vi "GUI.Config Test prueba con desplazador.vi"(11 "Path Config file":path) -> (3 "Path out":path)   [LabVIEW 2009]
uses:
  test.test de configuracion gui.ctl
  Test.ctl
  TEST.TEST CONFIG HW.ctl
  Rigol DP832/DP832_Control Channels.ctl
  TEST.TEST CONFIG TEST MATRIZ.ctl
  TEST.TEST CONFIG TEST.ctl
  TEST.TEST RESULT.ctl
  test_result fvasic.ctl
  TEST.TEST EXECUTION TEST.ctl
  TEST.TEST CONFIG VGA.ctl
  TEST.TEST TEST INFO.ctl
  TEST.TEST INFO PC.ctl
  machine estate configs.ctl
  Rigol DP832/DP832_Control Behavior.ctl
panel:
  out "FT_Handle":u32
  in  "Test":T1={"Config HW"={"VISA Rigol DP832"="Rigol_DP832", "Config Rigol DP832"=[{"Channel"=0, "V Limit"=5.5, "I Limit"=0.5, "V Out"=5.0}, {"Channel"=1, "V Limit"=5.5, "I Limit"=0.8, "V Out"=5.0}, {"Channel"=2, "V Limit"=5.5, "I Limit"=0.2, "V Out"=0.0}], "CTA Test#"="CTA013 A", "FT_Handle"=0, "Espera acceso FT"=10}, "Config Test"=[{"Vasic"=2.8, "Test Register?"=FALSE, "Test ADC?"=FALSE, "Test ADC"={"Repeats ADC"=100, "Max Desviation"=0.1}, "Limits ADC"={"Low"=[1.9, 1.3, 0.65, 0.0, 1.6, 1.4, 1.4, 0.9, 2.1, 0.85, 1.9], "High"=[2.1, 1.5, 0.85, 0.1, 1.4, 1.2, 1.2, 0.7, 1.9, 0.65, 1.7]}, "Test Max PN Min NP?"=FALSE, "Limits Max PN Min NP"={"Max P Upper"=1.888, "Min P Upper"=2.177000045776367, "Max N Upper"=0.818, "Min N Upper"=0.73, "Max P Lower"=1.475, "Min P Lower "=1.322, "Max N Lower"=1.321, "Min N Lower"=1.474}, "Test Rate Scan?"=FALSE, "Vin Rate Scan"=[], "Limits Rate Scan"={"High"=[0.15, 0.242, 0.331, 0.425, 0.512, 0.6, 0.688, 0.774, 0.847, 0.91], "Low"=[0.021, 0.11, 0.189, 0.27, 0.347, 0.421, 0.487, 0.551, 0.601, 0.635]}, "Test Rate Scan Adders?"=FALSE, "Vin Rate Adders"=[], "Test offset analog?"=FALSE, "Test offset digital?"=FALSE, "Lim Offset Analog"={"Max Analog"=0.05, "Min Analog"=-0.05}, "Lim offset Dig"={"Max Dig"=0.05}, "Limits Rate Scan adders"={"High"=[], "Low"=[]}}, {"Vasic"=2.8, "Test Register?"=FALSE, "Test ADC?"=FALSE, "Test ADC"={"Repeats ADC"=100, "Max Desviation"=0.1}, "Limits ADC"={"Low"=[1.9, 1.3, 0.65, 0.0, 1.6, 1.4, 1.4, 0.9, 2.1, 0.85, 1.9], "High"=[2.1, 1.5, 0.85, 0.1, 1.4, 1.2, 1.2, 0.7, 1.9, 0.65, 1.7]}, "Test Max PN Min NP?"=FALSE, "Limits Max PN Min NP"={"Max P Upper"=1.888, "Min P Upper"=2.177000045776367, "Max N Upper"=0.818, "Min N Upper"=0.73, "Max P Lower"=1.475, "Min P Lower "=1.322, "Max N Lower"=1.321, "Min N Lower"=1.474}, "Test Rate Scan?"=FALSE, "Vin Rate Scan"=[], "Limits Rate Scan"={"High"=[0.15, 0.242, 0.331, 0.425, 0.512, 0.6, 0.688, 0.774, 0.847, 0.91], "Low"=[0.021, 0.11, 0.189, 0.27, 0.347, 0.421, 0.487, 0.551, 0.601, 0.635]}, "Test Rate Scan Adders?"=FALSE, "Vin Rate Adders"=[], "Test offset analog?"=FALSE, "Test offset digital?"=FALSE, "Lim Offset Analog"={"Max Analog"=0.05, "Min Analog"=-0.05}, "Lim offset Dig"={"Max Dig"=0.05}, "Limits Rate Scan adders"={"High"=[], "Low"=[]}}, {"Vasic"=2.8, "Test Register?"=FALSE, "Test ADC?"=FALSE, "Test ADC"={"Repeats ADC"=100, "Max Desviation"=0.1}, "Limits ADC"={"Low"=[1.9, 1.3, 0.65, 0.0, 1.6, 1.4, 1.4, 0.9, 2.1, 0.85, 1.9], "High"=[2.1, 1.5, 0.85, 0.1, 1.4, 1.2, 1.2, 0.7, 1.9, 0.65, 1.7]}, "Test Max PN Min NP?"=FALSE, "Limits Max PN Min NP"={"Max P Upper"=1.888, "Min P Upper"=2.177000045776367, "Max N Upper"=0.818, "Min N Upper"=0.73, "Max P Lower"=1.475, "Min P Lower "=1.322, "Max N Lower"=1.321, "Min N Lower"=1.474}, "Test Rate Scan?"=FALSE, "Vin Rate Scan"=[], "Limits Rate Scan"={"High"=[0.15, 0.242, 0.331, 0.425, 0.512, 0.6, 0.688, 0.774, 0.847, 0.91], "Low"=[0.021, 0.11, 0.189, 0.27, 0.347, 0.421, 0.487, 0.551, 0.601, 0.635]}, "Test Rate Scan Adders?"=FALSE, "Vin Rate Adders"=[], "Test offset analog?"=FALSE, "Test offset digital?"=FALSE, "Lim Offset Analog"={"Max Analog"=0.05, "Min Analog"=-0.05}, "Lim offset Dig"={"Max Dig"=0.05}, "Limits Rate Scan adders"={"High"=[], "Low"=[]}}, {"Vasic"=2.8, "Test Register?"=FALSE, "Test ADC?"=FALSE, "Test ADC"={"Repeats ADC"=100, "Max Desviation"=0.1}, "Limits ADC"={"Low"=[1.9, 1.3, 0.65, 0.0, 1.6, 1.4, 1.4, 0.9, 2.1, 0.85, 1.9], "High"=[2.1, 1.5, 0.85, 0.1, 1.4, 1.2, 1.2, 0.7, 1.9, 0.65, 1.7]}, "Test Max PN Min NP?"=FALSE, "Limits Max PN Min NP"={"Max P Upper"=1.888, "Min P Upper"=2.177000045776367, "Max N Upper"=0.818, "Min N Upper"=0.73, "Max P Lower"=1.475, "Min P Lower "=1.322, "Max N Lower"=1.321, "Min N Lower"=1.474}, "Test Rate Scan?"=FALSE, "Vin Rate Scan"=[], "Limits Rate Scan"={"High"=[0.15, 0.242, 0.331, 0.425, 0.512, 0.6, 0.688, 0.774, 0.847, 0.91], "Low"=[0.021, 0.11, 0.189, 0.27, 0.347, 0.421, 0.487, 0.551, 0.601, 0.635]}, "Test Rate Scan Adders?"=FALSE, "Vin Rate Adders"=[], "Test offset analog?"=FALSE, "Test offset digital?"=FALSE, "Lim Offset Analog"={"Max Analog"=0.05, "Min Analog"=-0.05}, "Lim offset Dig"={"Max Dig"=0.05}, "Limits Rate Scan adders"={"High"=[], "Low"=[]}}], "Result"=[], "Execucion Test"={"Vasic Actual"=0}, "Config VGA"={"Theoretical Voltage"=[0.1, 0.2, 0.3, 0.4, 0.5, 0.6, 0.7, 0.8, 0.9, 1.0], "Real Voltage"=[0.10285, 0.20714, 0.29957, 0.40485, 0.49571, 0.60685, 0.69771, 0.80114, 0.89714, 0.99885], "Pulse Width"=57344, "Frecuency Pulse"=1000000.0, "VGA Gain"=[9, 16, 24, 34, 43, 52, 61, 72, 81, 93]}, "Test Info"={"Asic"="", "Operator"="", "Place"="", "Time start"=timestamp(0 s since 1904-01-01), "Time stop"=timestamp(0 s since 1904-01-01)}, "Info machine"={"SO"="", "SO Name"="", "SO Ver"="", "SO Build"="", "CPU"="", "APP"="", "APP YEAR"="", "APP ver"="", "APP User"="", "APP Serail"="", "MAC"=[], "PC NAME"=[], "PC IP"=[], "BIOS MANU"="", "BIOS NAME"="", "BIOS SERIAL"="", "BOARD MANU"="", "BOARD NAME"="", "BOARD SERIAL"="", "Driver Version"="", "Library Version"=""}} {"Config VGA"."Theoretical Voltage" format="%1.4f"; "Config VGA"."VGA Gain" format="%02x"; "Config VGA"."Frecuency Pulse" format="%0_2p"; "Config VGA"."Pulse Width" format="%04x"; "Config VGA"."Real Voltage" format="%1.5f"; "Config Test"."Limits Rate Scan adders"."Low" format="%1.3f"; "Config Test"."Limits Rate Scan adders"."High" format="%1.3f"; "Config Test"."Limits ADC"."High" format="%1.4f"; "Config Test"."Limits ADC"."Low" format="%1.3f"; "Config Test"."Lim offset Dig"."Max Dig" format="%.3g"; "Config Test"."Lim Offset Analog"."Min Analog" format="%.3g"; "Config Test"."Lim Offset Analog"."Max Analog" format="%.3g"; "Config Test"."Limits Rate Scan"."Low" format="%1.4f"; "Config Test"."Limits Rate Scan"."High" format="%1.3f"; "Config Test"."Limits Max PN Min NP"."Min P Upper" format="%.3g"; "Config Test"."Limits Max PN Min NP"."Min P Lower" format="%.3g"; "Config Test"."Limits Max PN Min NP"."Max N Lower" format="%.3g"; "Config Test"."Limits Max PN Min NP"."Max N Upper" format="%.3g"; "Config Test"."Limits Max PN Min NP"."Min N Lower" format="%.3g"; "Config Test"."Limits Max PN Min NP"."Min N Upper" format="%.3g"; "Config Test"."Limits Max PN Min NP"."Max P Upper" format="%.3g"; "Config Test"."Limits Max PN Min NP"."Max P Lower" format="%.3g"; "Config Test"."Vasic" min=2.8 max=3.8 step=0.01 format="%.2g"; "Config HW"."Config Rigol DP832"."Channel" items=["+30V Channel 1", "+30V Channel 2", "+5V Channel 3"]; "Config HW"."Config Rigol DP832"."V Limit" format="%.1g"; "Config HW"."Config Rigol DP832"."I Limit" format="%.1g"; "Config HW"."Config Rigol DP832"."V Out" format="%.1g"; "Result"."Test Registros"."Read W/R" format="%04x"; "Result"."Test Registros"."Pattern W/R" format="%04x"; "Result"."Test Registros"."Read Default" format="%04x"; "Result"."Test Registros"."Pattern Default" format="%04x"}
  in  "visualize":enum32{"Page 1", "Page 2"}(tab)
  in  "Elemensts":i32(listbox)
  in  "vga test":T12={"FRECUENCY PULSE"=-0.05, "PULSE WIDTH"=0, "CODE GAIN TEST"=0} {"CODE GAIN TEST" max=127 step=1; "PULSE WIDTH" format="%04x"; "FRECUENCY PULSE" format="%.3p"}
  in  "CTA Board":string(combo)
  in  "CHECK vga":bool
  in  "CHECK cta":bool
  in  "CHECK POWER":bool
  in  "Config Rigol DP832":T13(array[cluster])=[{"Channel"=0, "V Limit"=5.5, "I Limit"=0.5, "V Out"=5.0}, {"Channel"=1, "V Limit"=5.5, "I Limit"=0.8, "V Out"=5.0}, {"Channel"=2, "V Limit"=5.5, "I Limit"=0.2, "V Out"=0.0}] {"Channel" items=["+30V Channel 1", "+30V Channel 2", "+5V Channel 3"]; "V Limit" min=0.0 max=6.0 step=0.1 format="%.1g"; "I Limit" min=0.0 max=1.0 step=0.1 format="%.1g"; "V Out" min=0.0 max=6.0 step=0.1 format="%.1g"}
  in  "copy to new":bool
  in  "new":bool
  in  "delete":bool
  in  "TEST#":i32
  in  "VGA":T14={"VALUES VGA"=[], "TIME VGA"={"PULSE WIDTH"=0, "FRECUENCY PULSE"=-0.05}} {"TIME VGA"."FRECUENCY PULSE" format="%.3p"; "TIME VGA"."PULSE WIDTH" format="%04x"}
  in  "Valores":T15[](array[typedef])=[{"VOLTAGE SUPPLY ASIC"=2.5, "TEST ADC"=FALSE, "SETUP ADC 2"={"NUMBER OF REPETITIONS"=0, "MAX DESVIATION ADC"=-0.05}, "LIMITS MEASUREMENT ADC"=[], "TEST MAX MIN P/N"=FALSE, "LIMITS MAX PN MIN NP"=[], "TEST RATE SCAN"=FALSE, "VIN ASIC"=[], "LIMITS RATE SCAN"=[], "TEST RATE SCAN ADDERS"=FALSE, "VIN ASIC ADD"=[], "LIMITS RATE SCAN ADDERS"=[], "TEST OFFSET ANALOG"=FALSE, "LIMITS OFFSET ANALOG"={"MAXIMUM"=0.05, "MINIMUM"=-0.05}, "TEST OFFSET DIGITAL"=FALSE, "LIMITS OFFSET DIGITAL"={"MAXIMUM"=0.05}, "TEST REGISTER"=FALSE}] {"VOLTAGE SUPPLY ASIC" min=2.5 max=3.5 step=0.1 format="%.2g"; "LIMITS OFFSET DIGITAL"."MAXIMUM" format="%.3g"; "LIMITS OFFSET ANALOG"."MINIMUM" format="%.3g"; "LIMITS OFFSET ANALOG"."MAXIMUM" format="%.3g"; "SETUP ADC 2"."MAX DESVIATION ADC" format="%.3g"}
  in  "default":bool
  in  "Load config":bool
  in  "save config":bool
  in  "QUIT":bool
  in  "VISA Rigol DP832":refnum<visa-resource-name>="Rigol_DP832"
  # "Modo 2\nModo 3\nModo 4\nModo 2\nModo 3\nModo 4"
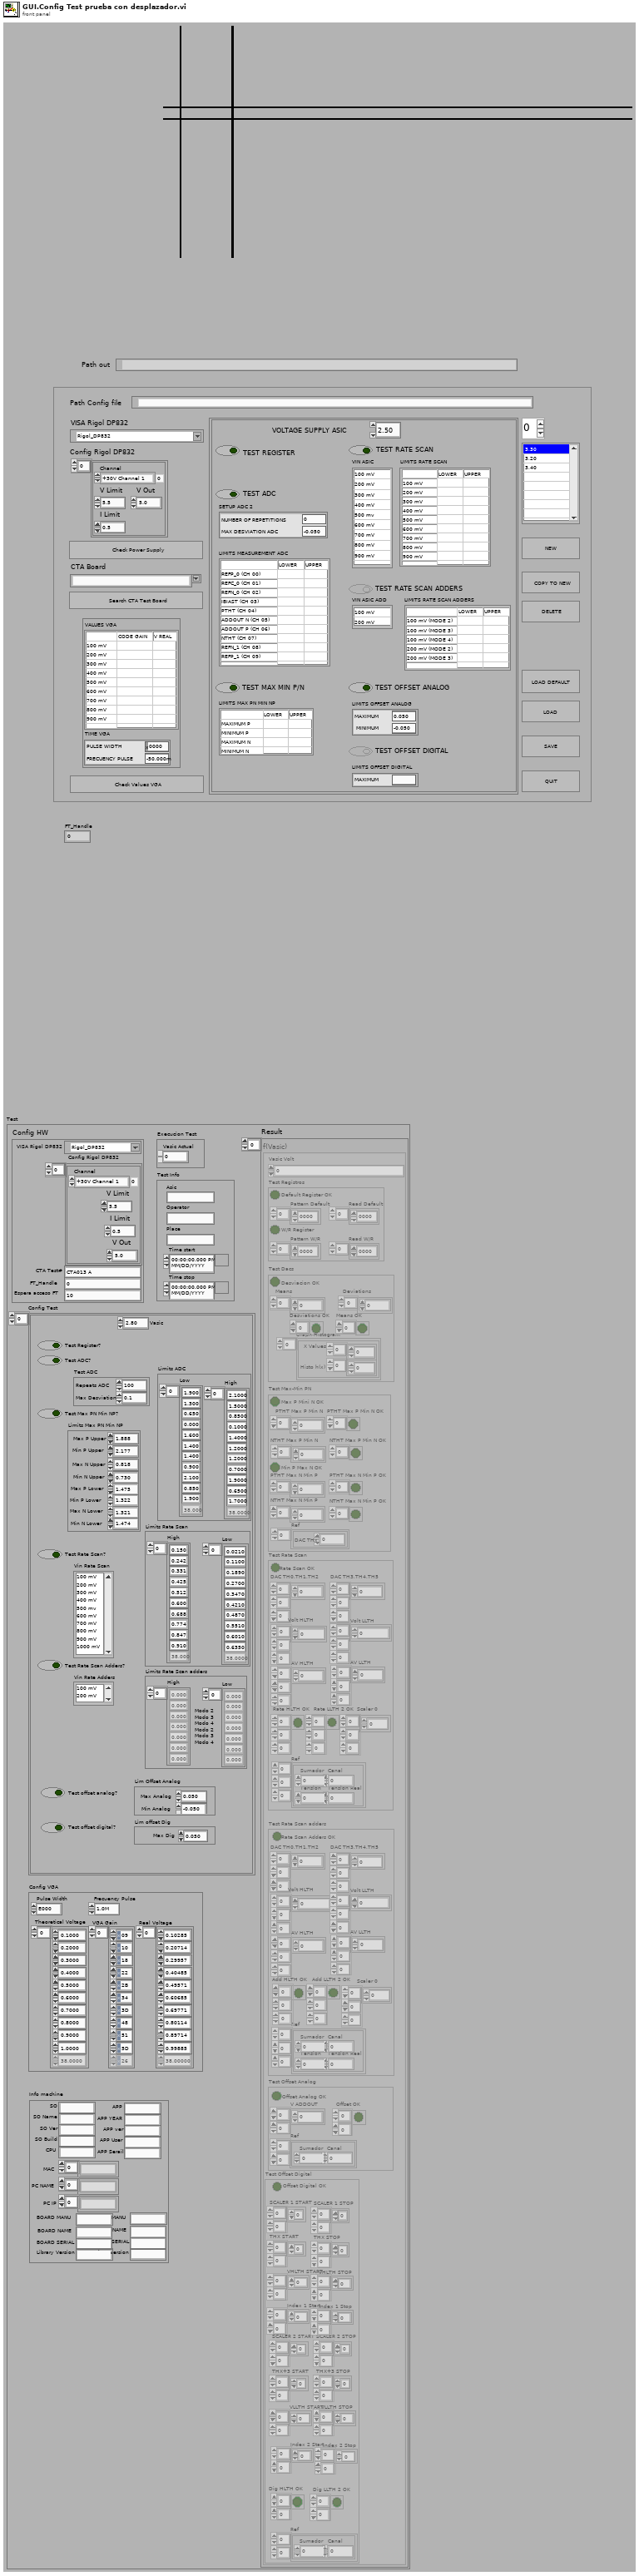
[diagram p1: front panel]
types:
  T1 = typedef "Test.ctl" = cluster{"Config HW":T2, "Config Test":T4, "Result":T6, "Execucion Test":T8, "Config VGA":T9, "Test Info":T10, "Info machine":T11}
  T2 = typedef "TEST.TEST CONFIG HW.ctl" = cluster{"VISA Rigol DP832":refnum<visa-resource-name>, "Config Rigol DP832":cluster{"Channel":T3, "V Limit":dbl, "I Limit":dbl, "V Out":dbl}[], "CTA Test#":string, "FT_Handle":u32, "Espera acceso FT":u32}
  T3 = typedef "DP832_Control Channels.ctl" = i32
  T4 = typedef "TEST.TEST CONFIG TEST MATRIZ.ctl" = T5[]
  T5 = typedef "TEST.TEST CONFIG TEST.ctl" = cluster{"Vasic":dbl, "Test Register?":bool, "Test ADC?":bool, "Test ADC":cluster{"Repeats ADC":i32, "Max Desviation":dbl}, "Limits ADC":cluster{"Low":dbl[], "High":dbl[]}, "Test Max PN Min NP?":bool, "Limits Max PN Min NP":cluster{"Max P Upper":dbl, "Min P Upper":dbl, "Max N Upper":dbl, "Min N Upper":dbl, "Max P Lower":dbl, "Min P Lower ":dbl, "Max N Lower":dbl, "Min N Lower":dbl}, "Test Rate Scan?":bool, "Vin Rate Scan":i32[], "Limits Rate Scan":cluster{"High":dbl[], "Low":dbl[]}, "Test Rate Scan Adders?":bool, "Vin Rate Adders":i32[], "Test offset analog?":bool, "Test offset digital?":bool, "Lim Offset Analog":cluster{"Max Analog":dbl, "Min Analog":dbl}, "Lim offset Dig":cluster{"Max Dig":dbl}, "Limits Rate Scan adders":cluster{"High":dbl[], "Low":dbl[]}}
  T6 = typedef "TEST.TEST RESULT.ctl" = T7[]
  T7 = typedef "test_result fvasic.ctl" = cluster{"Vasic Volt":i32, "Test Registros":cluster{"Default Register OK":bool, "Pattern Default":u16[], "Read Default":u16[], "W/R Register":bool, "Pattern W/R":u16[], "Read W/R":u16[]}, "Test Dacs":cluster{"Desviacion OK":bool, "Means":dbl[], "Deviations":dbl[], "Desviations OK":bool[], "Means OK":bool[], "Graph Histogram":cluster{"X Values":dbl[], "Histo h(x)":i32[]}[]}, "Test Max-Min PN":cluster{"Max P Mini N OK":bool, "PTHT Max P Min N":dbl[], "PTHT Max P Min N OK":bool[], "NTHT Max P Min N":dbl[], "NTHT Max P Min N OK":bool[], "Min P Max N OK":bool, "PTHT Max N Min P":dbl[], "PTHT Max N Min P OK":bool[], "NTHT Max N Min P":dbl[], "NTHT Max N Min P OK":bool[], "Ref":cluster{"DAC THx":u8}[]}, "Test Rate Scan":cluster{"Rate Scan OK":bool, "DAC TH0,TH1,TH2":u16[][][], "Volt HLTH":dbl[][][], "AV HLTH":dbl[][][], "Rate HLTH OK":bool[][][], "DAC TH3,TH4,TH5":u16[][][], "Volt LLTH":dbl[][][], "AV LLTH":dbl[][][], "Rate LLTH 2 OK":bool[][][], "Scaler 0":u16[][][], "Ref":cluster{"Sumador":u8, "Canal":u8, "Tension":u8, "Tension Real":dbl}[][][]}, "Test Rate Scan adders":cluster{"Rate Scan Adders OK":bool, "DAC TH0,TH1,TH2":u16[][][], "Volt HLTH":dbl[][][], "AV HLTH":dbl[][][], "Add HLTH OK":bool[][][], "DAC TH3,TH4,TH5":u16[][][], "Volt LLTH":dbl[][][], "AV LLTH":dbl[][][], "Add LLTH 2 OK":bool[][][], "Scaler 0":u16[][][], "Ref":cluster{"Sumador":u8, "Canal":u8, "Tension":u8, "Tension Real":dbl}[][][]}, "Test Offset Analog":cluster{"Offset Analog OK":bool, "V ADDOUT":dbl[][], "Offset OK":bool[][], "Ref":cluster{"Sumador":u8, "Canal":u8}[][]}, "Test Offset Digital":cluster{"Offset Digital OK":bool, "SCALER 1 START":u16[][], "SCALER 1 STOP":u16[][], "THX START":u16[][], "THX STOP":u16[][], "VHLTH START":dbl[][], "VHLTH STOP":dbl[][], "Index 1 Start":i32[][], "index 1 Stop":i32[][], "SCALER 2 START":u16[][], "SCALER 2 STOP":u16[][], "THX+3 START":u16[][], "THX+3 STOP":u16[][], "VLLTH START":dbl[][], "VLLTH STOP":dbl[][], "Index 2 Start":i32[][], "index 2 Stop":i32[][], "Dig HLTH OK":bool[][], "Dig LLTH 2 OK":bool[][], "Ref":cluster{"Sumador":u8, "Canal":u8}[][]}}
  T8 = typedef "TEST.TEST EXECUTION TEST.ctl" = cluster{"Vasic Actual":i32}
  T9 = typedef "TEST.TEST CONFIG VGA.ctl" = cluster{"Theoretical Voltage":dbl[], "Real Voltage":dbl[], "Pulse Width":u16, "Frecuency Pulse":dbl, "VGA Gain":u8[]}
  T10 = typedef "TEST.TEST TEST INFO.ctl" = cluster{"Asic":string, "Operator":string, "Place":string, "Time start":timestamp, "Time stop":timestamp}
  T11 = typedef "TEST.TEST INFO PC.ctl" = cluster{"SO":string, "SO Name":string, "SO Ver":string, "SO Build":string, "CPU":string, "APP":string, "APP YEAR":string, "APP ver":string, "APP User":string, "APP Serail":string, "MAC":string[], "PC NAME":string[], "PC IP":string[], "BIOS MANU":string, "BIOS NAME":string, "BIOS SERIAL":string, "BOARD MANU":string, "BOARD NAME":string, "BOARD SERIAL":string, "Driver Version":string, "Library Version":string}
  T12 = cluster{"FRECUENCY PULSE":dbl, "PULSE WIDTH":u16, "CODE GAIN TEST":u8}
  T13 = cluster{"Channel":T3, "V Limit":dbl, "I Limit":dbl, "V Out":dbl}[]
  T14 = cluster{"VALUES VGA":string[][], "TIME VGA":cluster{"PULSE WIDTH":u16, "FRECUENCY PULSE":dbl}}
  T15 = typedef "test.test de configuracion gui.ctl" = cluster{"VOLTAGE SUPPLY ASIC":dbl, "TEST ADC":bool, "SETUP ADC 2":cluster{"NUMBER OF REPETITIONS":i32, "MAX DESVIATION ADC":dbl}, "LIMITS MEASUREMENT ADC":string[][], "TEST MAX MIN P/N":bool, "LIMITS MAX PN MIN NP":string[][], "TEST RATE SCAN":bool, "VIN ASIC":i32[], "LIMITS RATE SCAN":string[][], "TEST RATE SCAN ADDERS":bool, "VIN ASIC ADD":i32[], "LIMITS RATE SCAN ADDERS":string[][], "TEST OFFSET ANALOG":bool, "LIMITS OFFSET ANALOG":cluster{"MAXIMUM":dbl, "MINIMUM":dbl}, "TEST OFFSET DIGITAL":bool, "LIMITS OFFSET DIGITAL":cluster{"MAXIMUM":dbl}, "TEST REGISTER":bool}
  T16 = typedef "machine estate configs.ctl" = enum16{"Init", "load init file", "wait", "Load File", "Refresh", "quit", "Save File", "Valores>Test", "Test>View", "quit save"}
  T17 = enum8{"Enabled", "Disabled", "Disabled and Grayed Out"}
  T18 = cluster{"VOLTAGE SUPPLY ASIC":dbl, "TEST ADC":bool, "SETUP ADC 2":cluster{"NUMBER OF REPETITIONS":i32, "MAX DESVIATION ADC":dbl}, "LIMITS MEASUREMENT ADC":string[][], "TEST MAX MIN P/N":bool, "LIMITS MAX PN MIN NP":string[][], "TEST RATE SCAN":bool, "VIN ASIC":i32[], "LIMITS RATE SCAN":string[][], "TEST RATE SCAN ADDERS":bool, "VIN ASIC ADD":i32[], "LIMITS RATE SCAN ADDERS":string[][], "TEST OFFSET ANALOG":bool, "LIMITS OFFSET ANALOG":cluster{"MAXIMUM":dbl, "MINIMUM":dbl}, "TEST OFFSET DIGITAL":bool, "LIMITS OFFSET DIGITAL":cluster{"MAXIMUM":dbl}, "TEST REGISTER":bool}[]
  T19 = cluster{"CTA Test#":string, "CTA Test#":string}[]
  T20 = cluster{"VISA Rigol DP832":refnum<visa-resource-name>, "CTA Test#":string}
  T21 = cluster{"Vsupply asic":dbl, "Test Register??":bool, "Test ADC??":bool, "Test ADC set":cluster{"Repeats ADC":i32, "Max Desviation":dbl}, "High ADC means":dbl[], "Low ADC means":dbl[], "Test MAX/MIN??":bool, "Limits Max PN Min NP":cluster{"Max P Lower":dbl, "Min P Lower ":dbl, "Max N Lower":dbl, "Min N Lower":dbl, "Max P Upper":dbl, "Min P Upper":dbl, "Min N Upper":dbl, "Max N Upper":dbl}, "Test rate scan":bool, "Vin Rate Scan":i32[], "High rate scan":dbl[], "Low rate scan":dbl[], "Test rate scan adders??":bool, "Vin Rate Adders":i32[], "High rate scan add":dbl[], "Low rate scan add":dbl[], "Test offset analog??":bool, "Lim Offset Analog":cluster{"Max Analog":dbl, "Min Analog":dbl}, "Test offset digital??":bool, "Lim offset Dig":cluster{"Max Dig":dbl}}[]
  T22 = typedef "DP832_Control Behavior.ctl" = u16
  T23 = cluster{"Device Index":u32, "FT_FLAGS_OPENED":bool, "FT_FLAGS_HISPEED":bool, "Type":u32, "VID":u32, "PID":u32, "LocID":i32, "Serial Number":string, "Description":string, "FT_Handle":u32}[]
  T24 = cluster{"Device Index":u32, "FT_FLAGS_OPENED":bool, "FT_FLAGS_HISPEED":bool, "Type":u32, "VID":u32, "PID":u32, "LocID":i32, "Serial Number":string, "Description":string, "FT_Handle":u32}
  T25 = cluster{"Serial Number":string, "Serial Number":string}
  T26 = cluster{"Vsupply asic":dbl, "Test Register??":bool, "Test ADC??":bool, "Test ADC set":cluster{"Repeats ADC":i32, "Max Desviation":dbl}, "High ADC means":dbl[], "Low ADC means":dbl[], "Test MAX/MIN??":bool, "Limits Max PN Min NP":cluster{"Max P Lower":dbl, "Min P Lower ":dbl, "Max N Lower":dbl, "Min N Lower":dbl, "Max P Upper":dbl, "Min P Upper":dbl, "Min N Upper":dbl, "Max N Upper":dbl}, "Test rate scan":bool, "Vin Rate Scan":i32[], "High rate scan":dbl[], "Low rate scan":dbl[], "Test rate scan adders??":bool, "Vin Rate Adders":i32[], "High rate scan add":dbl[], "Low rate scan add":dbl[], "Test offset analog??":bool, "Lim Offset Analog":cluster{"Max Analog":dbl, "Min Analog":dbl}, "Test offset digital??":bool, "Lim offset Dig":cluster{"Max Dig":dbl}}
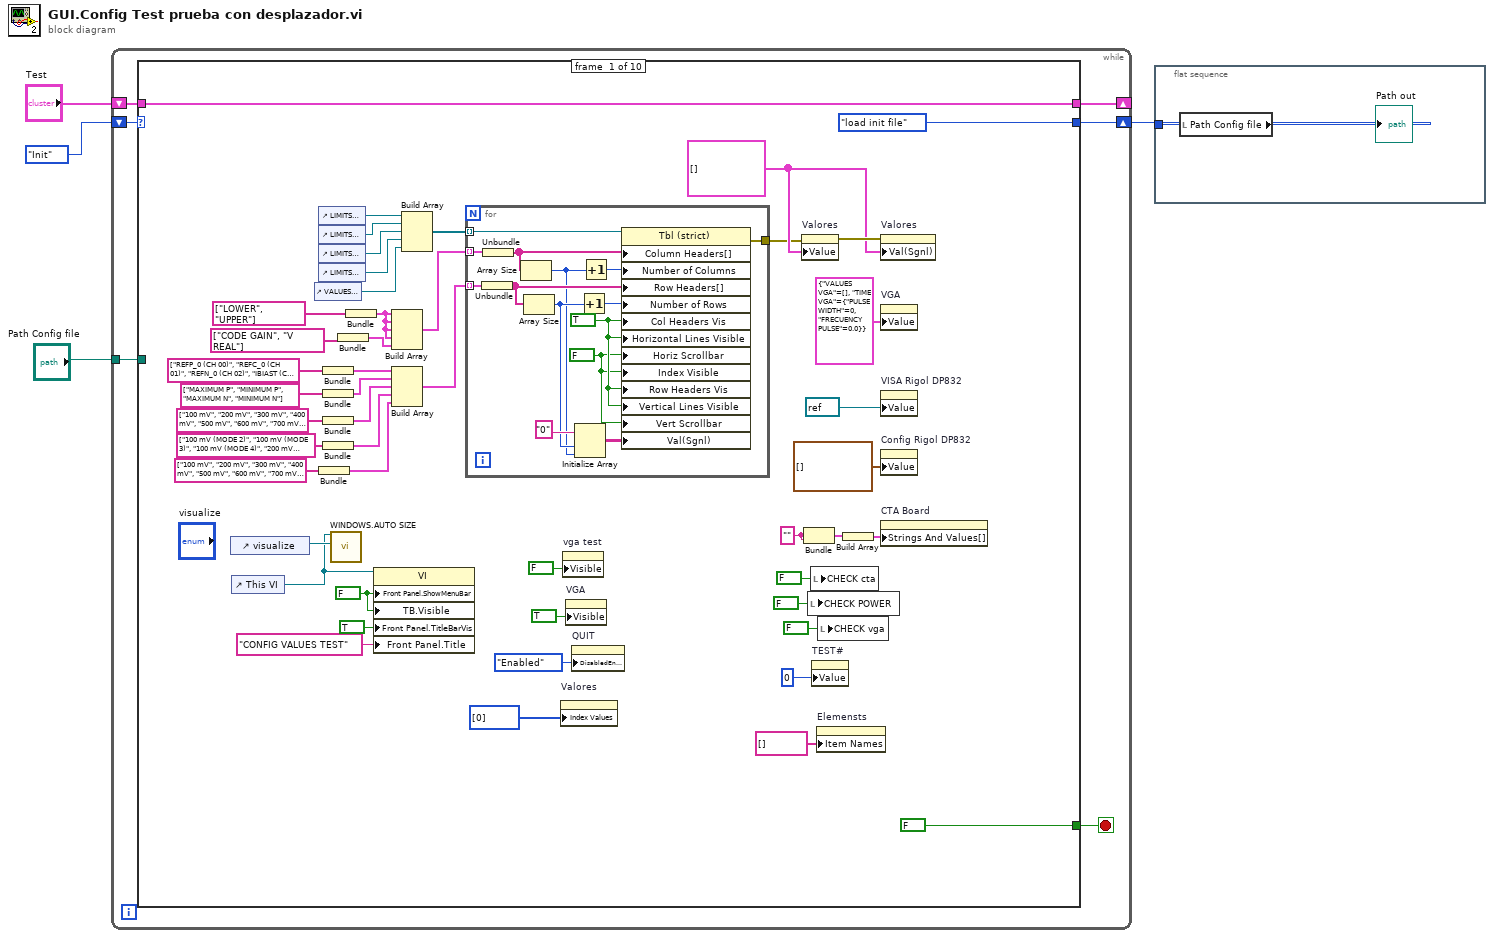
[diagram p0: block diagram]
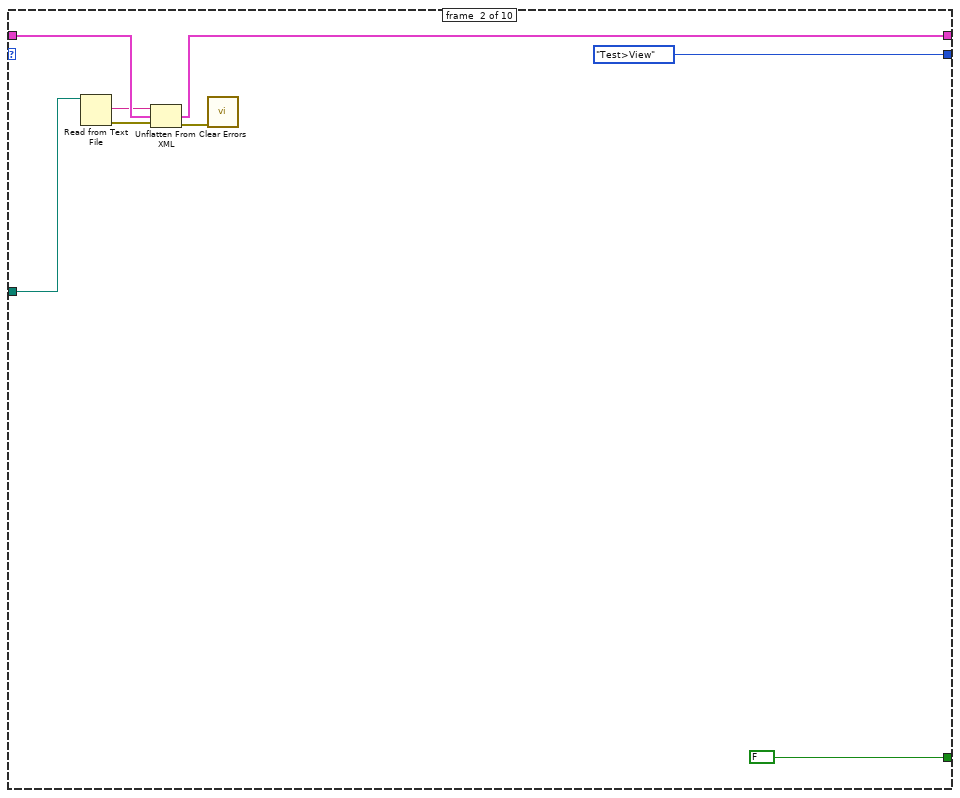
[diagram p2: hidden frame]
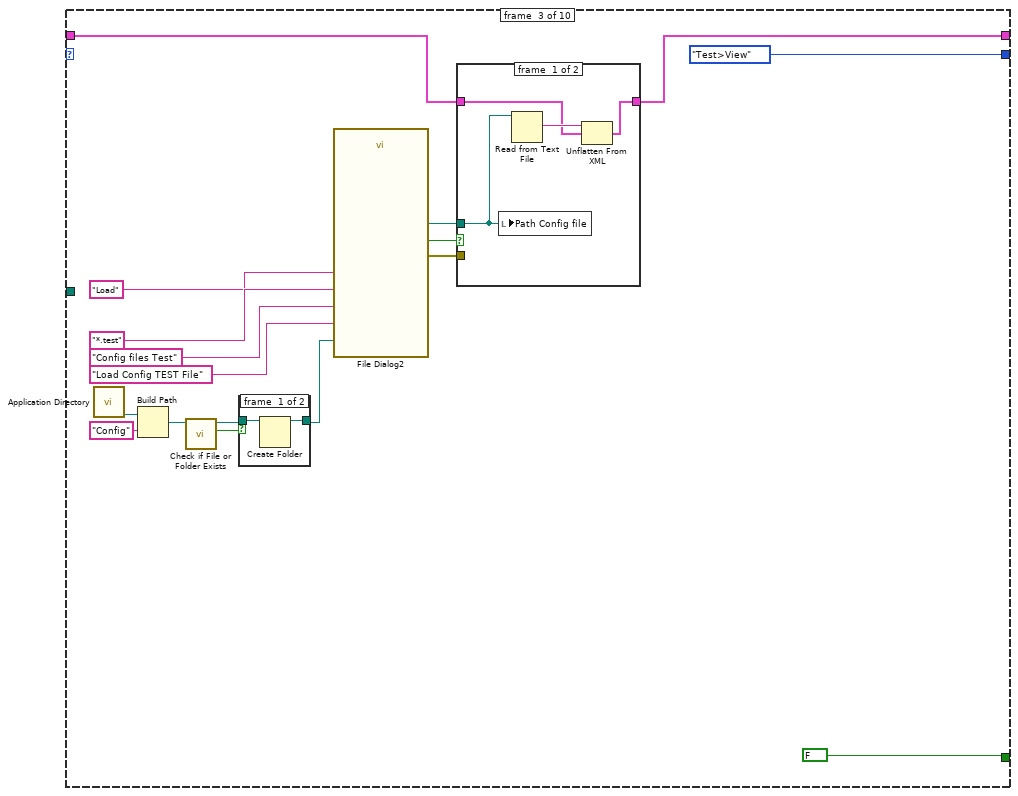
[diagram p3: hidden frame]
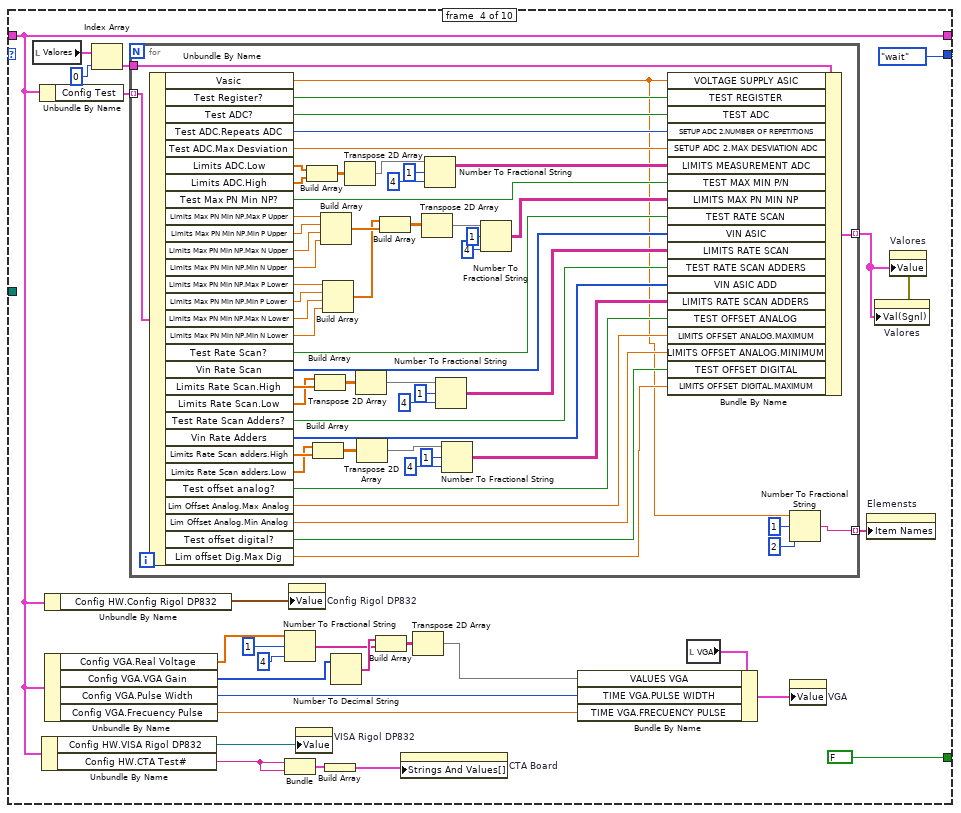
[diagram p6: hidden frame]
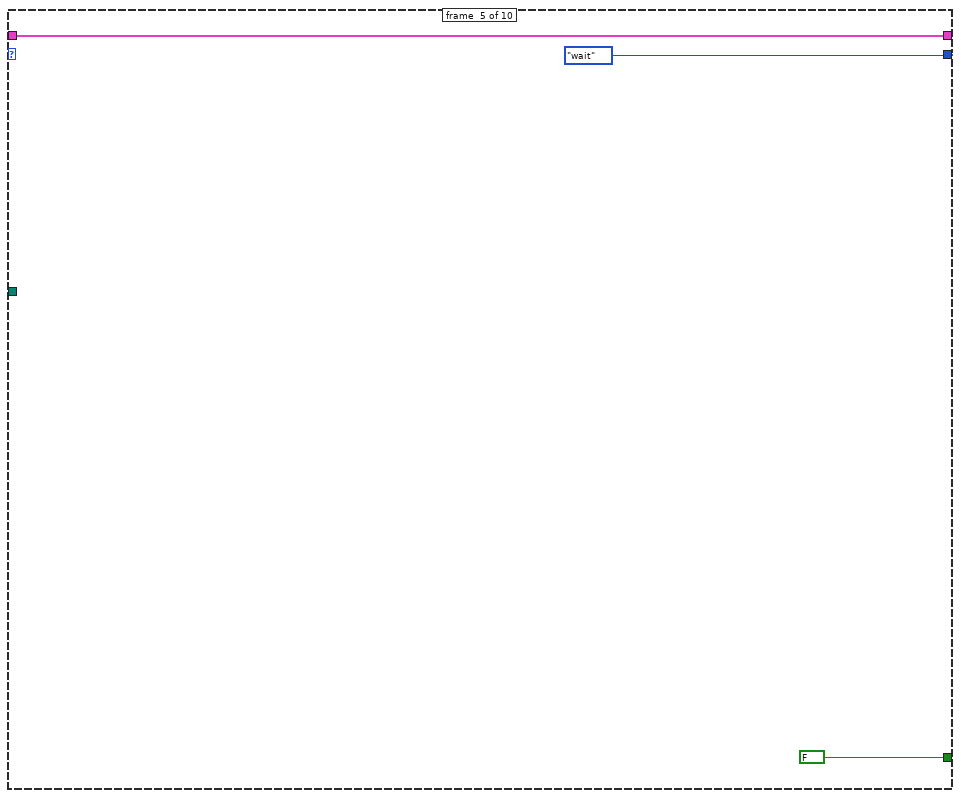
[diagram p7: hidden frame]
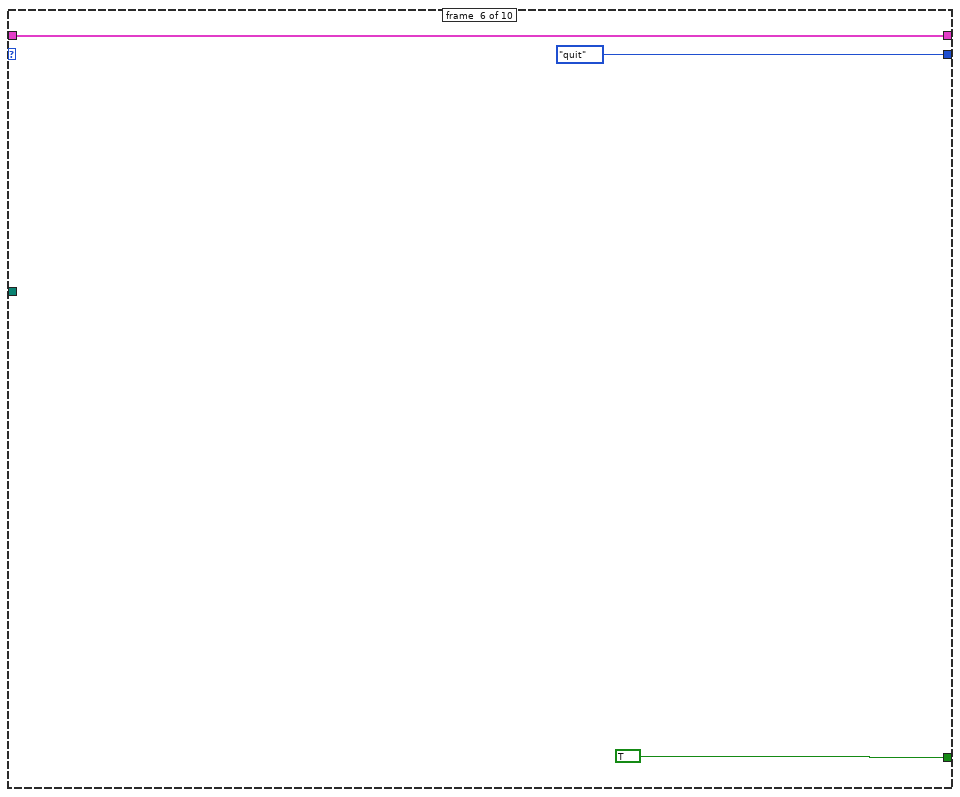
[diagram p8: hidden frame]
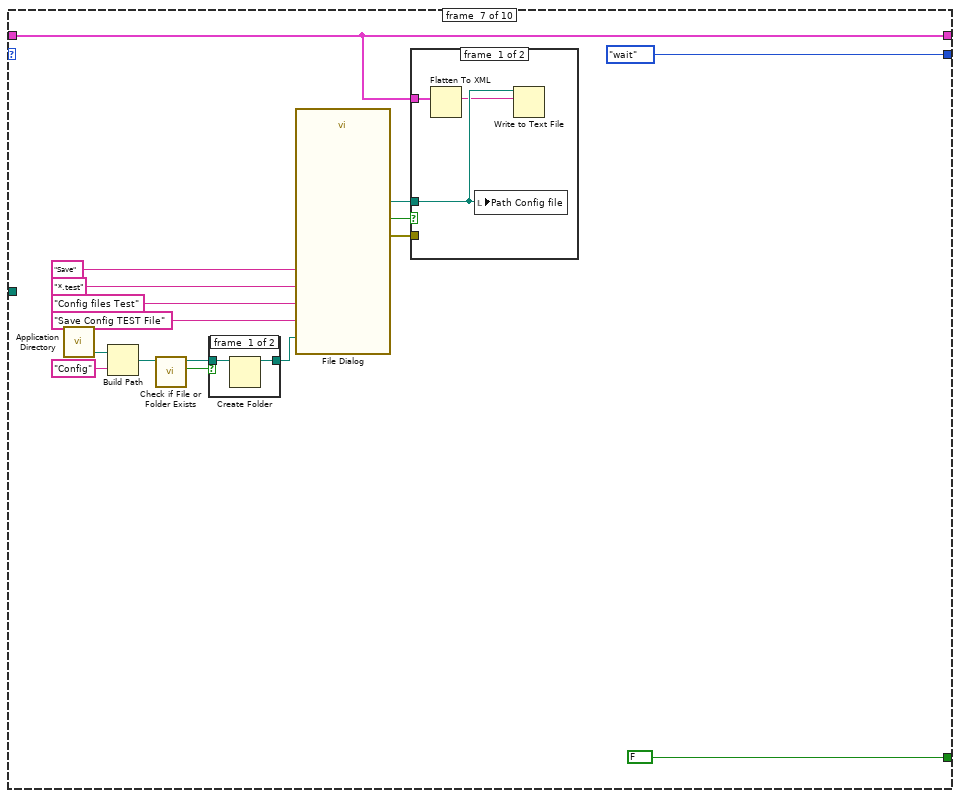
[diagram p9: hidden frame]
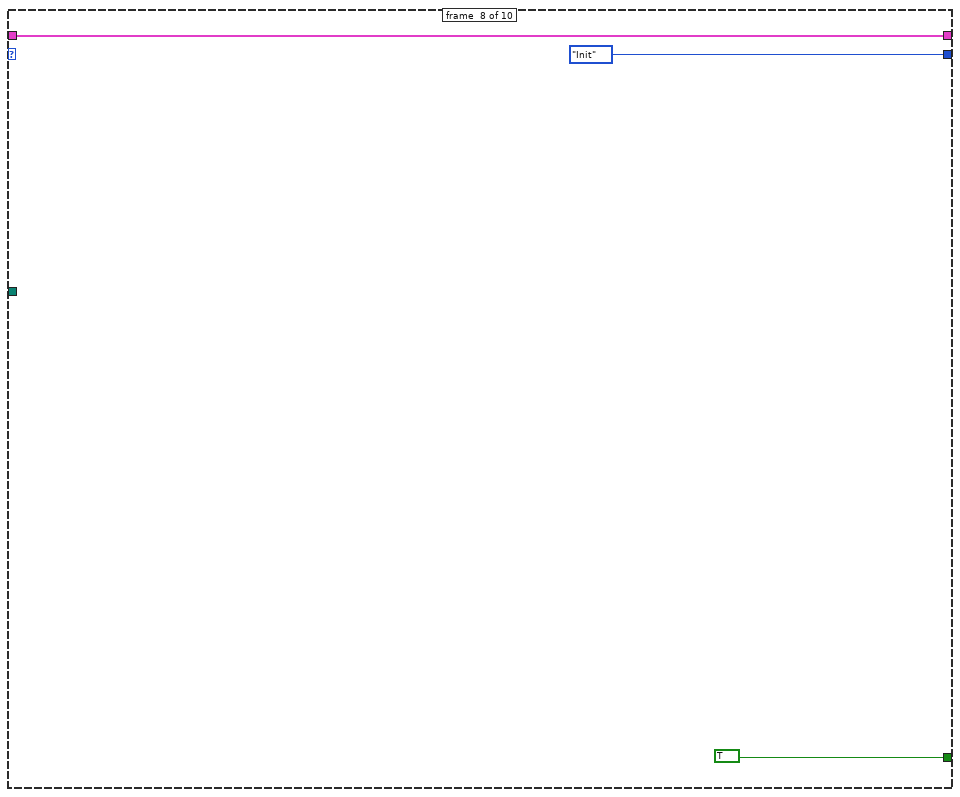
[diagram p12: hidden frame]
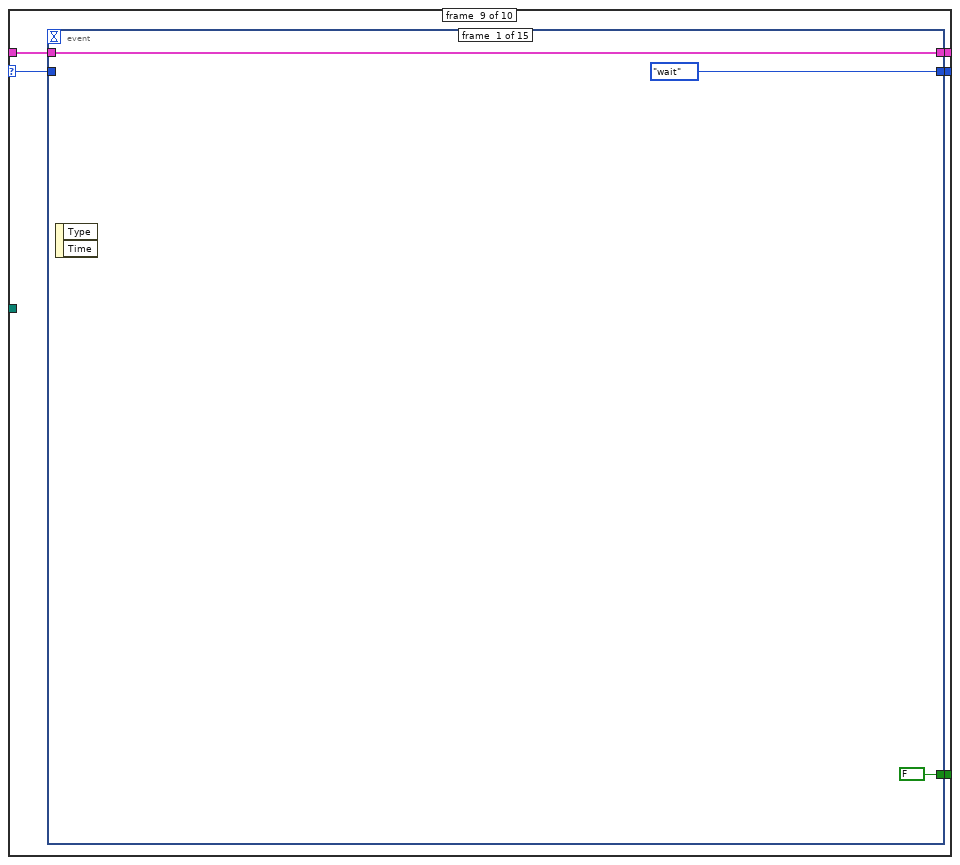
[diagram p13: hidden frame]
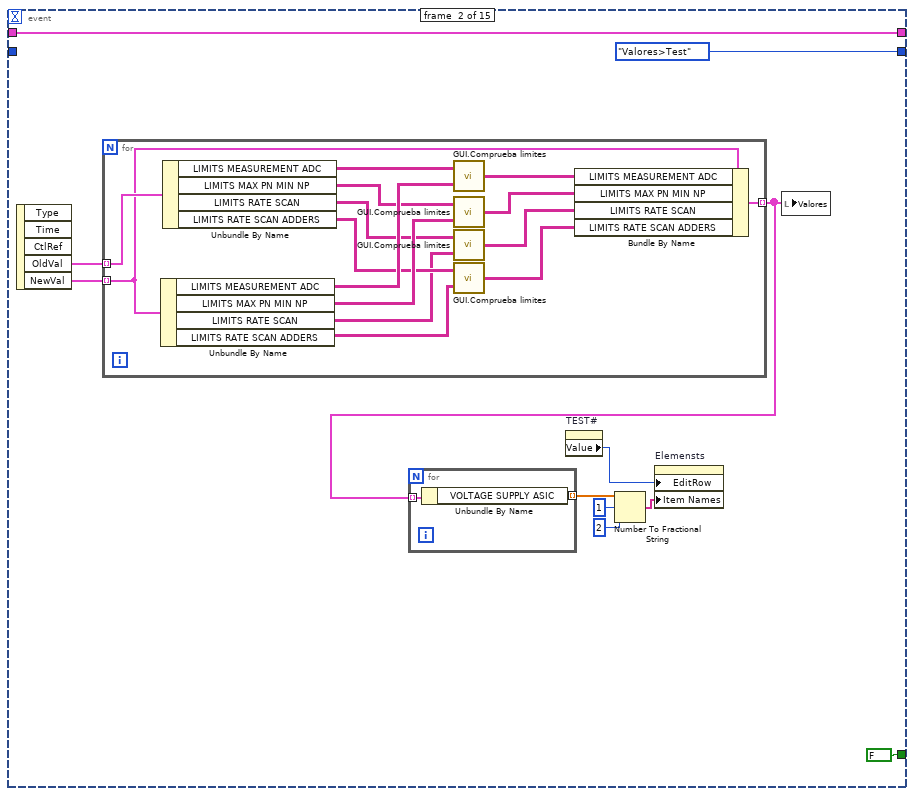
[diagram p14: hidden frame]
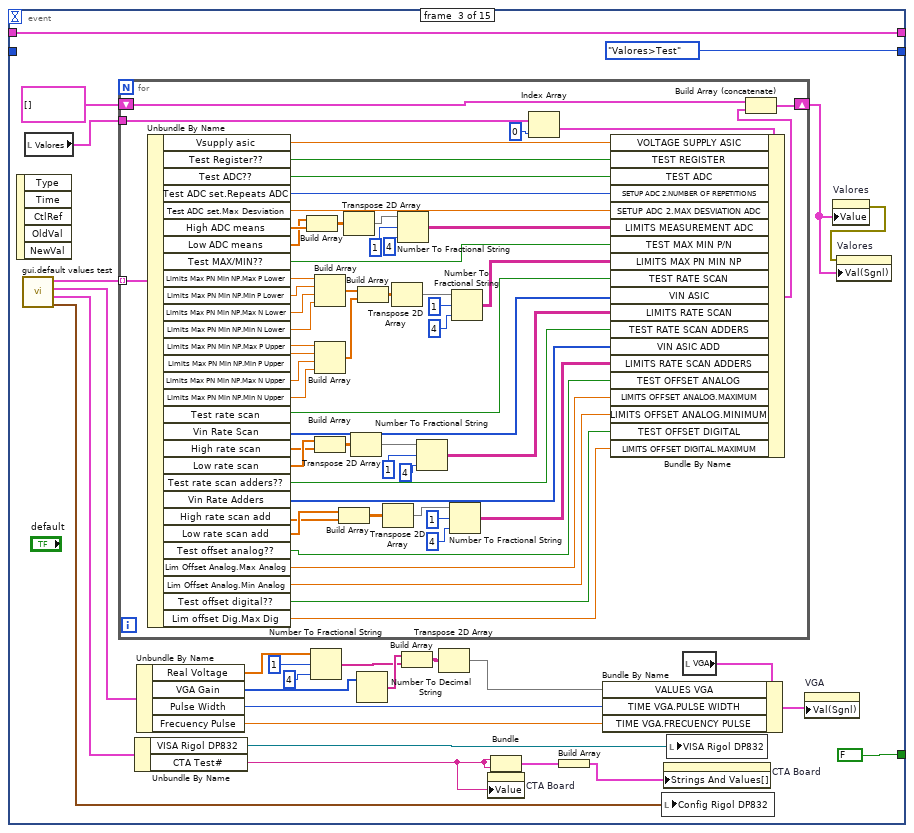
[diagram p15: hidden frame]
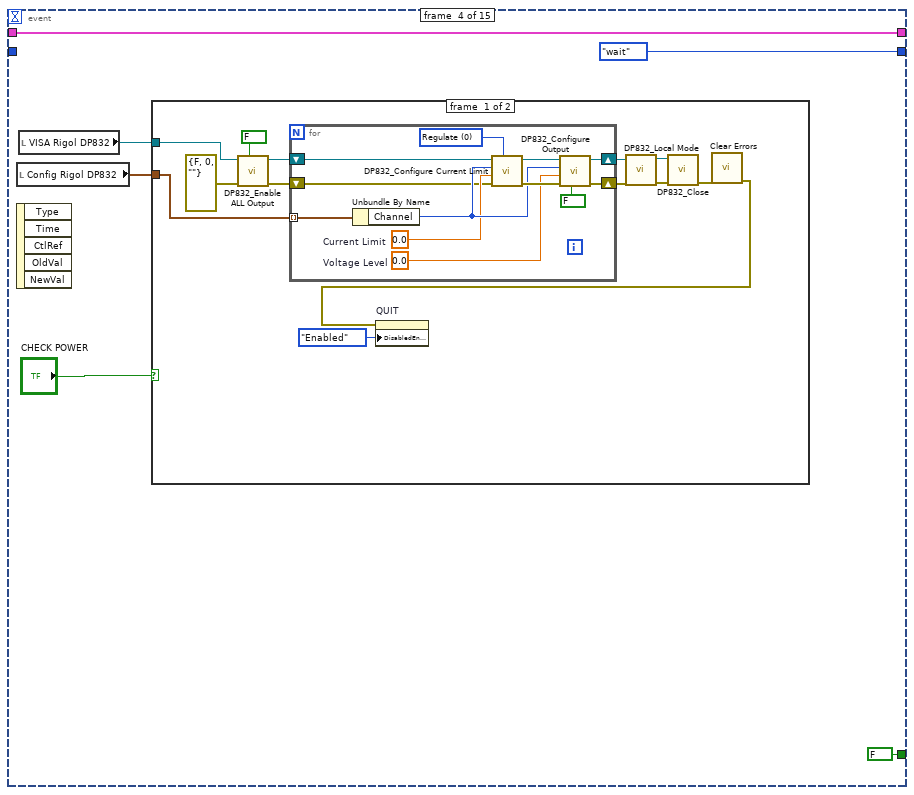
[diagram p16: hidden frame]
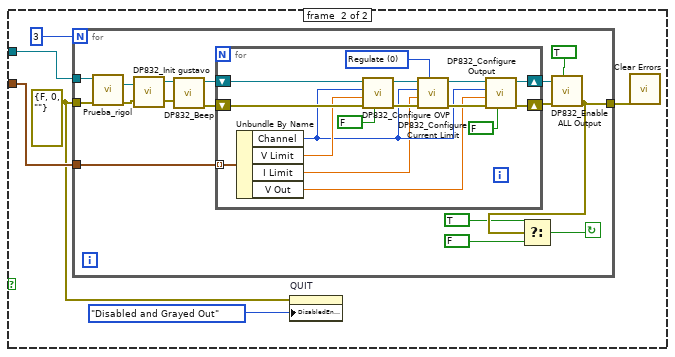
[diagram p17: hidden frame]
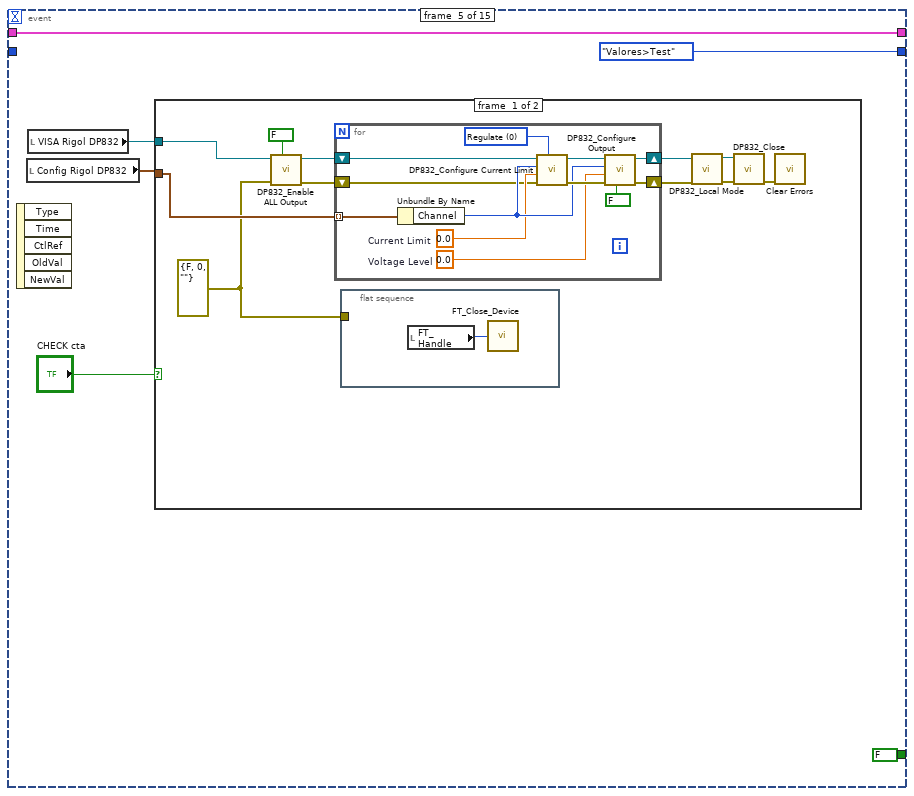
[diagram p18: hidden frame]
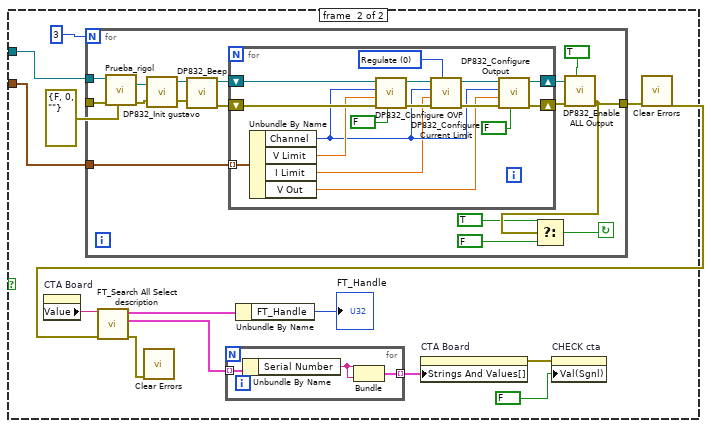
[diagram p19: hidden frame]
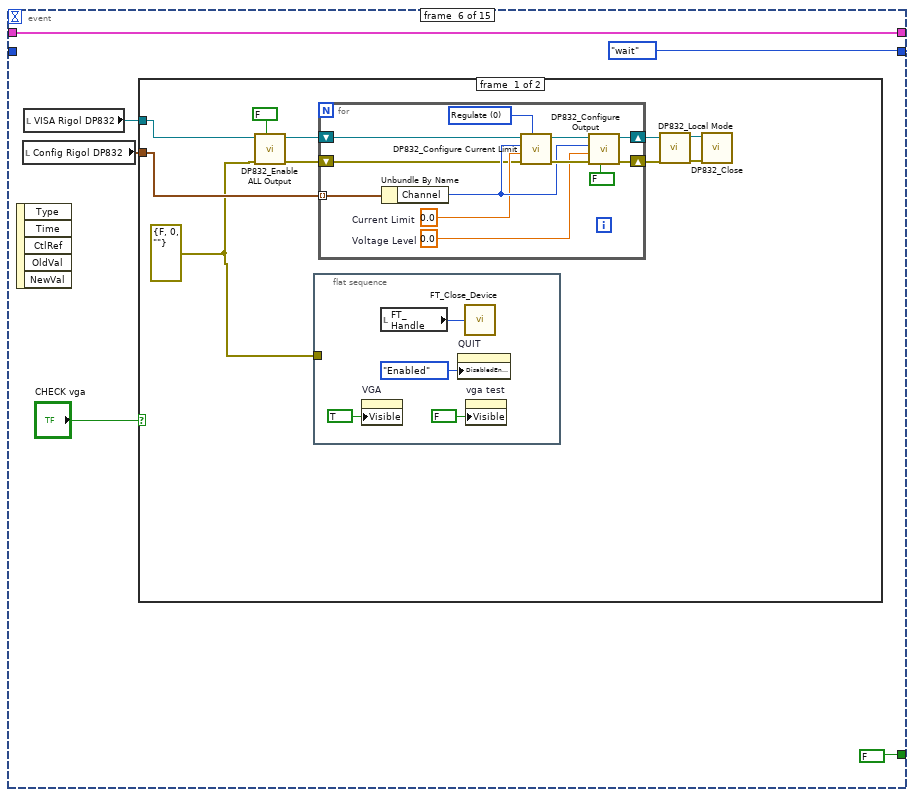
[diagram p20: hidden frame]
diagram:
  n1 = while {
    shift-right: [w8] -> w1
    shift-left: machine_estate_configs."Init" ("MACHINE") -> [w9]
    shift-right: [w6] -> _
    shift-left: "Test" -> [w7]
    tunnel: "Path Config file" -> [w5]
    stop <- w10 stop-if-true
    n2 = case shown="\"wait\"" w9 {
      selector: w9 -> [_ _ _ _ _ _ _ _ w224 _]
      tunnel: [FALSE FALSE FALSE FALSE FALSE TRUE FALSE TRUE w225 FALSE] -> w10
      tunnel: [machine_estate_configs."load init file" ("MACHINE") machine_estate_configs."Test>View" ("MACHINE") machine_estate_configs."Test>View" ("MACHINE") machine_estate_configs."wait" ("MACHINE") machine_estate_configs."wait" ("MACHINE") machine_estate_configs."quit" ("MACHINE") machine_estate_configs."wait" ("MACHINE") machine_estate_configs."Init" ("MACHINE") w223 machine_estate_configs."wait" ("MACHINE")] -> w8
      tunnel: [w29 w79 w82 w111 w190 w193 w196 w218 w221 w821] -> w6
      tunnel: w7 -> [w29 w80 w83 w111 w190 w193 w196 w218 w222 w822]
      tunnel: w5 -> [_ w75 _ _ _ _ _ _ _ _]
      frame #0 {
        w25 = T15[] [] ("Valores")
        w19 = "" ("CTA Test#")
        w41 = FALSE ("Front Panel Window:Show Menu Bar")
        n3 = control-ref of="visualize"() -> (w56:refnum<vi>)
        n4 = control-ref of="This VI"() -> (w38:refnum<vi>)
        n5 = control-ref of="VALUES VGA"() -> (w37:refnum<vi>)
        n6 = control-ref of="LIMITS MEASUREMENT ADC"() -> (w55:refnum<vi>)
        n7 = control-ref of="LIMITS MAX PN MIN NP"() -> (w54:refnum<vi>)
        n8 = control-ref of="LIMITS RATE SCAN"() -> (w53:refnum<vi>)
        n9 = control-ref of="LIMITS RATE SCAN ADDERS"() -> (w52:refnum<vi>)
        n10 = Bundle("Column Headers"=string[] ["100 mV", "200 mV", "300 mV", "400 mV", "500 mV", "600 mV", "700 mV", "800 mV", "900 mV", "1000 mV"]) -> (w32:cluster{"Column Headers":string[]})  [unwired: 1 in]
        n11 = Bundle("Column Headers"=string[] ["REFP_0 (CH 00)", "REFC_0 (CH 01)", "REFN_0 (CH 02)", "IBIAST (CH 03)", "PTHT (CH 04)", "ADDOUT N (CH 05)", "ADDOUT P (CH 06)", "NTHT (CH 07)", "REFN_1 (CH 08)", "REFP_1 (CH 09)", "VCOM (CH 10)"]) -> (w42:cluster{"Column Headers":string[]})  [unwired: 1 in]
        n12 = Bundle("Column Headers"=string[] ["MAXIMUM P", "MINIMUM P", "MAXIMUM N", "MINIMUM N"]) -> (w43:cluster{"Column Headers":string[]})  [unwired: 1 in]
        n13 = Bundle("Column Headers"=string[] ["100 mV", "200 mV", "300 mV", "400 mV", "500 mV", "600 mV", "700 mV", "800 mV", "900 mV", "1000 mV"]) -> (w44:cluster{"Column Headers":string[]})  [unwired: 1 in]
        n14 = Bundle("Column Headers"=string[] ["100 mV (MODE 2)", "100 mV (MODE 3)", "100 mV (MODE 4)", "200 mV (MODE 2)", "200 mV (MODE 3)", "200 mV (MODE 2)"]) -> (w45:cluster{"Column Headers":string[]})  [unwired: 1 in]
        n15 = call "WINDOWS.AUTO SIZE.vi"("TAB.AutoAjuste"=w56, "This VI"=w38) -> ()  [unwired: 5 in, 1 out]
        n16 = Bundle("Column Headers"=string[] ["CODE GAIN", "V REAL"]) -> (w30:cluster{"Column Headers":string[]})  [unwired: 1 in]
        n17 = Bundle("Column Headers"=string[] ["LOWER", "UPPER"]) -> (w35:cluster{"Column Headers":string[]})  [unwired: 1 in]
        n18 = property class="VI"(reference=w38, "Front Panel.ShowMenuBar"=w41, "TB.Visible"=w41, "Front Panel.TitleBarVis"=TRUE ("Front Panel Window:Title Bar Visible"), "Front Panel.Title"="CONFIG VALUES TEST" ("Front Panel Window:Title")) -> ()  [unwired: 1 in, 2 out]
        n19 = Build Array(w35, w35, w35, w35, w30) -> (w34:cluster{"Column Headers":string[]}[])
        n20 = Build Array(w42, w43, w44, w45, w32) -> (w50:cluster{"Column Headers":string[]}[])
        n21 = Build Array(w55, w54, w53, w52, w37) -> (w51:refnum<vi>[])
        n22 = for {
          tunnel: w34 -> [w61] mode=indexing
          tunnel: w50 -> [w62] mode=indexing
          tunnel: w51 -> [w68] mode=indexing
          tunnel: [w59] -> w22
          w69 = FALSE ("Autosizing Row Height")
          w70 = TRUE ("Autosizing Row Height")
          n23 = Unbundle(w62) -> ("Column Headers"=w67:string[])
          n24 = Unbundle(w61) -> ("Column Headers"=w60:string[])
          n25 = Array Size(array=w60) -> (size(s)=w63:i32)
          n26 = Array Size(array=w67) -> (size(s)=w65:i32)
          n27 = Initialize Array("0", w65, w63) -> (w64:string[][])
          n28 = Increment(x=w65) -> (x+1=w71:i32)
          n29 = Increment(x=w63) -> (x+1=w72:i32)
          n30 = property on="Property Node" class="Tbl (strict)"(reference=w68, "Column Headers[]"=w60, "Number of Columns"=w72, "Row Headers[]"=w67, "Number of Rows"=w71, "Col Headers Vis"=w70, "Horizontal Lines Visible"=w70, "Horiz Scrollbar"=w69, "Index Visible"=w69, "Row Headers Vis"=w70, "Vertical Lines Visible"=w70, "Vert Scrollbar"=w69, "Val(Sgnl)"=w64) -> (error out=w59:errorcluster)  [unwired: 1 in, 1 out]
        }
        n31 = property on="Valores" class="Arr (strict)"("Index Values"=u32[] [0]) -> ()  [unwired: 2 in, 2 out]
        n32 = property on="vga test" class="Clust (strict)"("Visible"=FALSE) -> ()  [unwired: 2 in, 2 out]
        n33 = property on="VGA" class="Clust (strict)"("Visible"=TRUE) -> ()  [unwired: 2 in, 2 out]
        n34 = property on="QUIT" class="Bool"("DisabledEnum"=T17."Enabled" ("Disabled")) -> ()  [unwired: 2 in, 2 out]
        n35 = property on="Valores" class="Arr (strict)"(error in=w22, "Value"=w25) -> (error out=w26:errorcluster)  [unwired: 1 in, 1 out]
        n36 = Bundle("CTA Test#"=w19, "CTA Test#"=w19) -> (w18:cluster{"CTA Test#":string, "CTA Test#":string})  [unwired: 1 in]
        n37 = local write "CHECK POWER"(FALSE ("CHECK POWER")) -> ()
        n38 = local write "CHECK cta"(FALSE ("CHECK cta")) -> ()
        n39 = property on="TEST#" class="DigNum (strict)"("Value"=0 ("Value (Signaling)")) -> ()  [unwired: 2 in, 2 out]
        n40 = property on="Elemensts" class="LstBox (strict)"("Item Names"=string[] []) -> ()  [unwired: 2 in, 2 out]
        n41 = local write "CHECK vga"(FALSE ("CHECK vga")) -> ()
        n42 = Build Array(w18) -> (w17:T19)
        n43 = property on="Valores" class="Arr (strict)"(error in=w26, "Val(Sgnl)"=w25) -> ()  [unwired: 1 in, 2 out]
        n44 = property on="VGA" class="Clust (strict)"("Value"=T14 {"VALUES VGA"=[], "TIME VGA"={"PULSE WIDTH"=0, "FRECUENCY PULSE"=0.0}} ("VGA")) -> ()  [unwired: 2 in, 2 out]
        n45 = property on="VISA Rigol DP832" class="VISAName"("Value"=refnum<visa-resource-name> refnum ("VISA Rigol DP832")) -> ()  [unwired: 2 in, 2 out]
        n46 = property on="Config Rigol DP832" class="Arr (strict)"("Value"=T13 [] ("Config Rigol DP832")) -> ()  [unwired: 2 in, 2 out]
        n47 = property on="CTA Board" class="CmbBox"("Strings And Values[]"=w17) -> ()  [unwired: 2 in, 2 out]
      }
      frame #1 {
        n48 = Read from Text File(file (use dialog)=w75) -> (text=w76:string, error out=w74:errorcluster)  [unwired: 3 in, 2 out]
        n49 = Unflatten From XML(xml string=w76, type=w80, error in (no error)=w74) -> (value=w79:T1, error out=w73:errorcluster)
        n50 = call <vilib>:"Clear Errors.vi"("error in (no error)"=w73) -> ()  [unwired: 6 in, 1 out]
      }
      frame #2 {
        n51 = call <vilib>:"Application Directory.vi"() -> ("Application Directory"=w86:path)
        n52 = Build Path(base path=w86, name or relative path="Config") -> (appended path=w93:path)
        n53 = call <vilib>:"Check if File or Folder Exists.vi"("path"=w93) -> ("file or folder exists?"=w85:bool, "dup path"=w92:path)  [unwired: 8 in, 1 out]
        n54 = case shown="False" w85 {
          tunnel: w92 -> [w104 w105]
          tunnel: [w103 w105] -> w81
          frame #0 {
            n55 = Create Folder(path (use dialog)=w104) -> (created path=w103:path)  [unwired: 2 in, 2 out]
          }
          frame #1 {
          }
        }
        n56 = call "File Dialog2"("start path"=w81, "prompt"="Load Config TEST File", "button label"="Load", "pattern (all files)"="*.test", "pattern label"="Config files Test") -> ("selected path"=w88:path, "cancelled"=w87:bool, "error out"=w84:errorcluster)  [unwired: 7 in, 1 out]
        n57 = case shown="False" w87 {
          tunnel: w88 -> [w98 _]
          tunnel: w84 -> [_ _]
          tunnel: [w99 w102] -> w82
          tunnel: w83 -> [w100 w102]
          frame #0 {
            n58 = local write "Path Config file"(w98) -> ()
            n59 = Read from Text File(file (use dialog)=w98) -> (text=w101:string)  [unwired: 3 in, 3 out]
            n60 = Unflatten From XML(xml string=w101, type=w100) -> (value=w99:T1)  [unwired: 1 in, 1 out]
          }
          frame #1 {
          }
        }
      }
      frame #3 {
        n61 = local read "Valores"() -> (w130:T15[])
        n62 = Unbundle By Name(w111) -> ("Config Test"=w127:T4)
        n63 = Unbundle By Name(w111) -> ("Config HW.VISA Rigol DP832"=w124:refnum<visa-resource-name>, "Config HW.CTA Test#"=w109:string)
        n64 = Unbundle By Name(w111) -> ("Config HW.Config Rigol DP832"=w110:T13)
        n65 = Unbundle By Name(w111) -> ("Config VGA.Real Voltage"=w115:dbl[], "Config VGA.VGA Gain"=w114:u8[], "Config VGA.Pulse Width"=w121:u16, "Config VGA.Frecuency Pulse"=w122:dbl)
        n66 = Index Array(array=w130, index=0) -> (element=w129:T15)
        n67 = for {
          tunnel: w129 -> [w189]
          tunnel: w127 -> [w188] mode=indexing
          tunnel: [w148] -> w125 mode=indexing
          tunnel: [w133] -> w106 mode=indexing
          n68 = Unbundle By Name(w188) -> ("Vasic"=w136:dbl, "Test Register?"=w147:bool, "Test ADC?"=w187:bool, "Test ADC.Repeats ADC"=w186:i32, "Test ADC.Max Desviation"=w185:dbl, "Limits ADC.Low"=w174:dbl[], "Limits ADC.High"=w173:dbl[], "Test Max PN Min NP?"=w184:bool, "Limits Max PN Min NP.Max P Upper"=w146:dbl, "Limits Max PN Min NP.Min P Upper"=w145:dbl, "Limits Max PN Min NP.Max N Upper"=w144:dbl, "Limits Max PN Min NP.Min N Upper"=w143:dbl, "Limits Max PN Min NP.Max P Lower"=w140:dbl, "Limits Max PN Min NP.Min P Lower"=w139:dbl, "Limits Max PN Min NP.Max N Lower"=w138:dbl, "Limits Max PN Min NP.Min N Lower"=w137:dbl, "Test Rate Scan?"=w166:bool, "Vin Rate Scan"=w165:i32[], "Limits Rate Scan.High"=w156:dbl[], "Limits Rate Scan.Low"=w155:dbl[], "Test Rate Scan Adders?"=w149:bool, "Vin Rate Adders"=w152:i32[], "Limits Rate Scan adders.High"=w154:dbl[], "Limits Rate Scan adders.Low"=w153:dbl[], "Test offset analog?"=w179:bool, "Lim Offset Analog.Max Analog"=w180:dbl, "Lim Offset Analog.Min Analog"=w181:dbl, "Test offset digital?"=w182:bool, "Lim offset Dig.Max Dig"=w183:dbl)
          n69 = Build Array(w174, w173) -> (w176:dbl[][])
          n70 = Build Array(w153, w154) -> (w159:dbl[][])
          n71 = Build Array(w155, w156) -> (w162:dbl[][])
          n72 = Build Array(w146, w145, w144, w143) -> (w142:dbl[])
          n73 = Build Array(w140, w139, w138, w137) -> (w141:dbl[])
          n74 = Transpose 2D Array(2D array=w176) -> (transposed array=w175:dbl[][])
          n75 = Transpose 2D Array(2D array=w162) -> (transposed array=w161:dbl[][])
          n76 = Transpose 2D Array(2D array=w159) -> (transposed array=w160:dbl[][])
          n77 = Build Array(w141, w142) -> (w170:dbl[][])
          n78 = Transpose 2D Array(2D array=w170) -> (transposed array=w171:dbl[][])
          n79 = Number To Fractional String(number=w175, width (-)=i16 1, precision (6)=i16 4) -> (F-format string=w172:string[][])  [unwired: 1 in]
          n80 = Number To Fractional String(number=w161, width (-)=i16 1, precision (6)=i16 4) -> (F-format string=w150:string[][])  [unwired: 1 in]
          n81 = Number To Fractional String(number=w160, width (-)=i16 1, precision (6)=i16 4) -> (F-format string=w151:string[][])  [unwired: 1 in]
          n82 = Number To Fractional String(number=w171, width (-)=i16 1, precision (6)=i16 4) -> (F-format string=w167:string[][])  [unwired: 1 in]
          n83 = Bundle By Name(cluster=w189, "VOLTAGE SUPPLY ASIC"=w136, "TEST REGISTER"=w147, "TEST ADC"=w187, "SETUP ADC 2.NUMBER OF REPETITIONS"=w186, "SETUP ADC 2.MAX DESVIATION ADC"=w185, "LIMITS MEASUREMENT ADC"=w172, "TEST MAX MIN P/N"=w184, "LIMITS MAX PN MIN NP"=w167, "TEST RATE SCAN"=w166, "VIN ASIC"=w165, "LIMITS RATE SCAN"=w150, "TEST RATE SCAN ADDERS"=w149, "VIN ASIC ADD"=w152, "LIMITS RATE SCAN ADDERS"=w151, "TEST OFFSET ANALOG"=w179, "LIMITS OFFSET ANALOG.MAXIMUM"=w180, "LIMITS OFFSET ANALOG.MINIMUM"=w181, "TEST OFFSET DIGITAL"=w182, "LIMITS OFFSET DIGITAL.MAXIMUM"=w183) -> (w148:T15)
          n84 = Number To Fractional String(number=w136, width (-)=i16 1, precision (6)=i16 2) -> (F-format string=w133:string)  [unwired: 1 in]
        }
        n85 = Number To Fractional String(number=w115, width (-)=i16 1, precision (6)=i16 4) -> (F-format string=w116:string[])  [unwired: 1 in]
        n86 = Bundle("CTA Test#"=w109, "CTA Test#"=w109) -> (w108:cluster{"CTA Test#":string, "CTA Test#":string})  [unwired: 1 in]
        n87 = property on="Config Rigol DP832" class="Arr (strict)"("Value"=w110) -> ()  [unwired: 2 in, 2 out]
        n88 = property on="VISA Rigol DP832" class="VISAName"("Value"=w124) -> ()  [unwired: 2 in, 2 out]
        n89 = Build Array(w108) -> (w107:T19)
        n90 = Number To Decimal String(number=w114) -> (decimal integer string=w117:string[])  [unwired: 1 in]
        n91 = Build Array(w117, w116) -> (w118:string[][])
        n92 = property on="CTA Board" class="CmbBox"("Strings And Values[]"=w107) -> ()  [unwired: 2 in, 2 out]
        n93 = Transpose 2D Array(2D array=w118) -> (transposed array=w113:string[][])
        n94 = local read "VGA"() -> (w123:T14)
        n95 = Bundle By Name(cluster=w123, "VALUES VGA"=w113, "TIME VGA.PULSE WIDTH"=w121, "TIME VGA.FRECUENCY PULSE"=w122) -> (w112:T14)
        n96 = property on="VGA" class="Clust (strict)"("Value"=w112) -> ()  [unwired: 2 in, 2 out]
        n97 = property on="Elemensts" class="LstBox (strict)"("Item Names"=w106) -> ()  [unwired: 2 in, 2 out]
        n98 = property on="Valores" class="Arr (strict)"("Value"=w125) -> (error out=w126:errorcluster)  [unwired: 2 in, 1 out]
        n99 = property on="Valores" class="Arr (strict)"(error in=w126, "Val(Sgnl)"=w125) -> ()  [unwired: 1 in, 2 out]
      }
      frame #4 {
      }
      frame #5 {
      }
      frame #6 {
        n100 = call <vilib>:"Application Directory.vi"() -> ("Application Directory"=w199:path)
        n101 = Build Path(base path=w199, name or relative path="Config") -> (appended path=w207:path)
        n102 = call <vilib>:"Check if File or Folder Exists.vi"("path"=w207) -> ("file or folder exists?"=w198:bool, "dup path"=w206:path)  [unwired: 8 in, 1 out]
        n103 = case shown="False" w198 {
          tunnel: w206 -> [w216 w217]
          tunnel: [w215 w217] -> w205
          frame #0 {
            n104 = Create Folder(path (use dialog)=w216) -> (created path=w215:path)  [unwired: 2 in, 2 out]
          }
          frame #1 {
          }
        }
        n105 = call "File Dialog"("start path"=w205, "prompt"="Save Config TEST File", "button label"="Save", "pattern (all files)"="*.test", "pattern label"="Config files Test") -> ("selected path"=w201:path, "cancelled"=w200:bool, "error out"=w197:errorcluster)  [unwired: 7 in, 1 out]
        n106 = case shown="False" w200 {
          tunnel: w201 -> [w214 _]
          tunnel: w197 -> [_ _]
          tunnel: w196 -> [w213 _]
          frame #0 {
            n107 = Flatten To XML(anything=w213) -> (xml string=w212:string)
            n108 = local write "Path Config file"(w214) -> ()
            n109 = Write to Text File(file (use dialog)=w214, text=w212) -> ()  [unwired: 2 in, 3 out]
          }
          frame #1 {
          }
        }
      }
      frame #7 {
      }
      frame #8 {
        n110 = event shown="[9] \"new\": Value Change" {
          selector: _ -> [_ _ _ _ _ _ _ _ _ _ _ _ _ _ _]
          dyn-events: _ -> [_ _ _ _ _ _ _ _ _ _ _ _ _ _ _]
          timeout: _ -> [_ _ _ _ _ _ _ _ _ _ _ _ _ _ _]
          tunnel: [FALSE FALSE FALSE FALSE FALSE FALSE FALSE FALSE _ FALSE FALSE FALSE FALSE TRUE FALSE] -> w225
          tunnel: w224 -> [_ _ _ _ _ _ _ _ _ _ _ _ _ _ _]
          tunnel: [machine_estate_configs."wait" ("MACHINE") machine_estate_configs."Valores>Test" ("MACHINE") machine_estate_configs."Valores>Test" ("MACHINE") machine_estate_configs."wait" ("MACHINE") machine_estate_configs."Valores>Test" ("MACHINE") machine_estate_configs."wait" ("MACHINE") machine_estate_configs."wait" ("MACHINE") machine_estate_configs."wait" ("MACHINE") _ machine_estate_configs."Valores>Test" ("MACHINE") machine_estate_configs."Load File" ("MACHINE") machine_estate_configs."wait" ("MACHINE") machine_estate_configs."wait" ("MACHINE") machine_estate_configs."wait" ("MACHINE") machine_estate_configs."Save File" ("MACHINE")] -> w223
          tunnel: w222 -> [w226 w235 w260 w346 w411 w489 w570 w586 _ w618 w685 w695 w709 w732 w755]
          tunnel: [w226 w235 w260 w346 w411 w489 w570 w586 _ w618 w685 w695 w709 w732 w738] -> w221
          event #0 {
            n111 = event-data() -> ()  [unwired: 1 in, 2 out]
          }
          event #1 {
            n112 = event-data() -> ("OldVal"=w236:T15[], "NewVal"=w237:T15[])  [unwired: 1 in, 3 out]
            n113 = for {
              tunnel: w237 -> [w245] mode=indexing
              tunnel: w236 -> [w256] mode=indexing
              tunnel: [w253] -> w230 mode=indexing
              n114 = Unbundle By Name(w245) -> ("LIMITS MEASUREMENT ADC"=w252:string[][], "LIMITS MAX PN MIN NP"=w250:string[][], "LIMITS RATE SCAN"=w246:string[][], "LIMITS RATE SCAN ADDERS"=w247:string[][])
              n115 = Unbundle By Name(w256) -> ("LIMITS MEASUREMENT ADC"=w255:string[][], "LIMITS MAX PN MIN NP"=w251:string[][], "LIMITS RATE SCAN"=w249:string[][], "LIMITS RATE SCAN ADDERS"=w248:string[][])
              n116 = call "GUI.Comprueba limites.vi"("LIMITS MEASUREMENT ADC"=w252, "LIMITS MEASUREMENT ADC 2"=w255) -> ("Array"=w254:string[][])
              n117 = call "GUI.Comprueba limites.vi"("LIMITS MEASUREMENT ADC"=w250, "LIMITS MEASUREMENT ADC 2"=w251) -> ("Array"=w244:string[][])
              n118 = call "GUI.Comprueba limites.vi"("LIMITS MEASUREMENT ADC"=w246, "LIMITS MEASUREMENT ADC 2"=w249) -> ("Array"=w243:string[][])
              n119 = call "GUI.Comprueba limites.vi"("LIMITS MEASUREMENT ADC"=w247, "LIMITS MEASUREMENT ADC 2"=w248) -> ("Array"=w242:string[][])
              n120 = Bundle By Name(cluster=w245, "LIMITS MEASUREMENT ADC"=w254, "LIMITS MAX PN MIN NP"=w244, "LIMITS RATE SCAN"=w243, "LIMITS RATE SCAN ADDERS"=w242) -> (w253:T15)
            }
            n121 = for {
              tunnel: [w241] -> w231 mode=indexing
              tunnel: w230 -> [w240] mode=indexing
              n122 = Unbundle By Name(w240) -> ("VOLTAGE SUPPLY ASIC"=w241:dbl)
            }
            n123 = property on="TEST#" class="DigNum (strict)"() -> ("Value"=w229:i32)  [unwired: 2 in, 2 out]
            n124 = Number To Fractional String(number=w231, width (-)=i16 1, precision (6)=i16 2) -> (F-format string=w232:string[])  [unwired: 1 in]
            n125 = property on="Elemensts" class="LstBox (strict)"("EditRow"=w229, "Item Names"=w232) -> ()  [unwired: 2 in, 2 out]
            n126 = local write "Valores"(w230) -> ()
          }
          event #2 {
            n127 = event-data() -> ()  [unwired: 1 in, 5 out]
            n128 = call "gui.default values test.vi"() -> ("Config Rigol DP832"=w262:T13, "Config Hw"=w279:T20, "Config VGA"=w280:T9, "Values default"=w281:T21)  [unwired: 8 in]
            n129 = local read "Valores"() -> (w282:T15[])
            n130 = for {
              tunnel: w282 -> [w341]
              tunnel: w281 -> [w339] mode=indexing
              shift-right: [w290] -> w266
              shift-left: T18 [] ("Valores") -> [w288]
              n131 = Unbundle By Name(w339) -> ("Vsupply asic"=w284:dbl, "Test Register??"=w287:bool, "Test ADC??"=w338:bool, "Test ADC set.Repeats ADC"=w337:i32, "Test ADC set.Max Desviation"=w336:dbl, "High ADC means"=w333:dbl[], "Low ADC means"=w332:dbl[], "Test MAX/MIN??"=w329:bool, "Limits Max PN Min NP.Max P Lower"=w328:dbl, "Limits Max PN Min NP.Min P Lower"=w327:dbl, "Limits Max PN Min NP.Max N Lower"=w326:dbl, "Limits Max PN Min NP.Min N Lower"=w325:dbl, "Limits Max PN Min NP.Max P Upper"=w295:dbl, "Limits Max PN Min NP.Min P Upper"=w294:dbl, "Limits Max PN Min NP.Max N Upper"=w293:dbl, "Limits Max PN Min NP.Min N Upper"=w292:dbl, "Test rate scan"=w319:bool, "Vin Rate Scan"=w318:i32[], "High rate scan"=w298:dbl[], "Low rate scan"=w299:dbl[], "Test rate scan adders??"=w313:bool, "Vin Rate Adders"=w312:i32[], "High rate scan add"=w296:dbl[], "Low rate scan add"=w297:dbl[], "Test offset analog??"=w307:bool, "Lim Offset Analog.Max Analog"=w306:dbl, "Lim Offset Analog.Min Analog"=w305:dbl, "Test offset digital??"=w304:bool, "Lim offset Dig.Max Dig"=w303:dbl)
              n132 = Build Array(w332, w333) -> (w331:dbl[][])
              n133 = Build Array(w328, w327, w326, w325) -> (w324:dbl[])
              n134 = Build Array(w295, w294, w293, w292) -> (w323:dbl[])
              n135 = Build Array(w299, w298) -> (w315:dbl[][])
              n136 = Build Array(w297, w296) -> (w311:dbl[][])
              n137 = Transpose 2D Array(2D array=w331) -> (transposed array=w302:dbl[][])
              n138 = Transpose 2D Array(2D array=w315) -> (transposed array=w301:dbl[][])
              n139 = Build Array(w324, w323) -> (w286:dbl[][])
              n140 = Transpose 2D Array(2D array=w311) -> (transposed array=w300:dbl[][])
              n141 = Transpose 2D Array(2D array=w286) -> (transposed array=w285:dbl[][])
              n142 = Number To Fractional String(number=w302, width (-)=i16 1, precision (6)=i16 4) -> (F-format string=w330:string[][])  [unwired: 1 in]
              n143 = Number To Fractional String(number=w301, width (-)=i16 1, precision (6)=i16 4) -> (F-format string=w314:string[][])  [unwired: 1 in]
              n144 = Number To Fractional String(number=w300, width (-)=i16 1, precision (6)=i16 4) -> (F-format string=w308:string[][])  [unwired: 1 in]
              n145 = Number To Fractional String(number=w285, width (-)=i16 1, precision (6)=i16 4) -> (F-format string=w320:string[][])  [unwired: 1 in]
              n146 = Index Array(array=w341, index=0) -> (element=w340:T15)
              n147 = Bundle By Name(cluster=w340, "VOLTAGE SUPPLY ASIC"=w284, "TEST REGISTER"=w287, "TEST ADC"=w338, "SETUP ADC 2.NUMBER OF REPETITIONS"=w337, "SETUP ADC 2.MAX DESVIATION ADC"=w336, "LIMITS MEASUREMENT ADC"=w330, "TEST MAX MIN P/N"=w329, "LIMITS MAX PN MIN NP"=w320, "TEST RATE SCAN"=w319, "VIN ASIC"=w318, "LIMITS RATE SCAN"=w314, "TEST RATE SCAN ADDERS"=w313, "VIN ASIC ADD"=w312, "LIMITS RATE SCAN ADDERS"=w308, "TEST OFFSET ANALOG"=w307, "LIMITS OFFSET ANALOG.MAXIMUM"=w306, "LIMITS OFFSET ANALOG.MINIMUM"=w305, "TEST OFFSET DIGITAL"=w304, "LIMITS OFFSET DIGITAL.MAXIMUM"=w303) -> (w289:T15)
              n148 = Build Array (concatenate)(w288, w289) -> (w290:T15[])
            }
            n149 = Unbundle By Name(w279) -> ("VISA Rigol DP832"=w263:refnum<visa-resource-name>, "CTA Test#"=w257:string)
            n150 = Unbundle By Name(w280) -> ("Real Voltage"=w273:dbl[], "VGA Gain"=w271:u8[], "Pulse Width"=w275:u16, "Frecuency Pulse"=w276:dbl)
            n151 = Number To Fractional String(number=w273, width (-)=i16 1, precision (6)=i16 4) -> (F-format string=w267:string[])  [unwired: 1 in]
            n152 = Number To Decimal String(number=w271) -> (decimal integer string=w268:string[])  [unwired: 1 in]
            n153 = Build Array(w268, w267) -> (w270:string[][])
            n154 = Transpose 2D Array(2D array=w270) -> (transposed array=w269:string[][])
            n155 = property on="CTA Board" class="CmbBox"("Value"=w257) -> ()  [unwired: 2 in, 2 out]
            n156 = Bundle("CTA Test#"=w257, "CTA Test#"=w257) -> (w259:cluster{"CTA Test#":string, "CTA Test#":string})  [unwired: 1 in]
            n157 = Build Array(w259) -> (w258:T19)
            n158 = local write "Config Rigol DP832"(w262) -> ()
            n159 = property on="CTA Board" class="CmbBox"("Strings And Values[]"=w258) -> ()  [unwired: 2 in, 2 out]
            n160 = local write "VISA Rigol DP832"(w263) -> ()
            n161 = local read "VGA"() -> (w278:T14)
            n162 = Bundle By Name(cluster=w278, "VALUES VGA"=w269, "TIME VGA.PULSE WIDTH"=w275, "TIME VGA.FRECUENCY PULSE"=w276) -> (w277:T14)
            n163 = property on="VGA" class="Clust (strict)"("Val(Sgnl)"=w277) -> ()  [unwired: 2 in, 2 out]
            n164 = property on="Valores" class="Arr (strict)"("Value"=w266) -> (error out=w265:errorcluster)  [unwired: 2 in, 1 out]
            n165 = property on="Valores" class="Arr (strict)"(error in=w265, "Val(Sgnl)"=w266) -> ()  [unwired: 1 in, 2 out]
          }
          event #3 {
            n166 = local read "Config Rigol DP832"() -> (w343:T13)
            n167 = event-data() -> ()  [unwired: 1 in, 5 out]
            n168 = local read "VISA Rigol DP832"() -> (w344:refnum<visa-resource-name>)
            n169 = case shown="False" "CHECK POWER" {
              tunnel: w344 -> [w353 w377]
              tunnel: w343 -> [w352 w376]
              frame #0 {
                n170 = call "DP832_Enable ALL Output.vi"("Enable Output (T: Enable)"=FALSE, "error in (no error)"=errorcluster {"status"=FALSE, "code"=0, "source"=""}, "VISA resource name"=w353) -> ("error out"=w358:errorcluster, "VISA resource name out"=w359:refnum<visa-resource-name>)  [unwired: 7 in]
                n171 = for {
                  shift-right: [w367] -> w354
                  shift-left: w358 -> [w363]
                  shift-right: [w368] -> w355
                  shift-left: w359 -> [w364]
                  tunnel: w352 -> [w362] mode=indexing
                  w361 = 0.0  # Voltage Level
                  w365 = 0.0  # Current Limit
                  w369 = T22 0 items=["Regulate", "Trip"] ("Behavior (0: Regulate)")
                  n172 = Unbundle By Name(w362) -> ("Channel"=w366:T3)
                  n173 = call "DP832_Configure Current Limit.vi"("Behavior"=w369, "error in (no error)"=w363, "Current Limit"=w365, "Channel"=w366, "VISA resource name"=w364) -> ("error out"=w371:errorcluster, "VISA resource name out"=w372:refnum<visa-resource-name>)  [unwired: 5 in]
                  n174 = call "DP832_Configure Output.vi"("Enable Output (T: Enable)"=FALSE, "error in (no error)"=w371, "Voltage Level"=w361, "Channel"=w366, "VISA resource name"=w372) -> ("error out"=w367:errorcluster, "VISA resource name out"=w368:refnum<visa-resource-name>)  [unwired: 5 in]
                }
                n175 = call "DP832_Local Mode.vi"("error in (no error)"=w354, "VISA resource name"=w355) -> ("error out"=w357:errorcluster, "VISA resource name out"=w356:refnum<visa-resource-name>)  [unwired: 8 in]
                n176 = call "DP832_Close.vi"("error in (no error)"=w357, "VISA resource name"=w356) -> ("error out"=w350:errorcluster)  [unwired: 8 in, 1 out]
                n177 = call <vilib>:"Clear Errors.vi"("error in (no error)"=w350) -> ("error out"=w348:errorcluster)  [unwired: 6 in]
                n178 = property on="QUIT" class="Bool"(error in=w348, "DisabledEnum"=T17."Enabled" ("Disabled")) -> ()  [unwired: 1 in, 2 out]
              }
              frame #1 {
                w373 = errorcluster {"status"=FALSE, "code"=0, "source"=""} ("error in")
                n179 = for {
                  N: 3 -> [_]
                  tunnel: [w382] -> w375
                  tunnel: w376 -> [w388]
                  tunnel: w377 -> [w385]
                  tunnel: w373 -> [w384]
                  stop <- w380 continue-if-true
                  n180 = call "Prueba_rigol.vi"("error in (no error)"=w384, "VISA IN"=w385) -> ("error out 2"=w383:errorcluster)  [unwired: 8 in, 1 out]
                  n181 = call "DP832_Init gustavo.vi"("error in (no error)"=w383, "VISA resource name 2"=w385) -> ("error out"=w386:errorcluster, "VISA resource name"=w387:refnum<visa-resource-name>)
                  n182 = call "DP832_Beep.vi"("error in (no error)"=w386, "VISA resource name"=w387) -> ("error out"=w392:errorcluster, "VISA resource name out"=w393:refnum<visa-resource-name>)  [unwired: 8 in]
                  n183 = for {
                    shift-right: [w399] -> w390
                    shift-left: w392 -> [w401]
                    shift-right: [w400] -> w391
                    shift-left: w393 -> [w402]
                    tunnel: w388 -> [w398] mode=indexing
                    w403 = T22 0 items=["Regulate", "Trip"] ("Behavior (0: Regulate)")
                    n184 = Unbundle By Name(w398) -> ("Channel"=w396:T3, "V Limit"=w397:dbl, "I Limit"=w395:dbl, "V Out"=w394:dbl)
                    n185 = call "DP832_Configure OVP.vi"("Enable OVP (T: Enable)"=FALSE, "error in (no error)"=w401, "Voltage Limit"=w397, "Channel"=w396, "VISA resource name"=w402) -> ("error out"=w406:errorcluster, "VISA resource name out"=w405:refnum<visa-resource-name>)  [unwired: 5 in]
                    n186 = call "DP832_Configure Current Limit.vi"("Behavior"=w403, "error in (no error)"=w406, "Current Limit"=w395, "Channel"=w396, "VISA resource name"=w405) -> ("error out"=w408:errorcluster, "VISA resource name out"=w409:refnum<visa-resource-name>)  [unwired: 5 in]
                    n187 = call "DP832_Configure Output.vi"("Enable Output (T: Enable)"=FALSE, "error in (no error)"=w408, "Voltage Level"=w394, "Channel"=w396, "VISA resource name"=w409) -> ("error out"=w399:errorcluster, "VISA resource name out"=w400:refnum<visa-resource-name>)  [unwired: 5 in]
                  }
                  n188 = call "DP832_Enable ALL Output.vi"("Enable Output (T: Enable)"=TRUE, "error in (no error)"=w390, "VISA resource name"=w391) -> ("error out"=w382:errorcluster)  [unwired: 7 in, 1 out]
                  n189 = Select(t=TRUE, s=w382, f=FALSE) -> (s? t:f=w380:bool)
                }
                n190 = property on="QUIT" class="Bool"(error in=w373, "DisabledEnum"=T17."Disabled and Grayed Out" ("Disabled")) -> ()  [unwired: 1 in, 2 out]
                n191 = call <vilib>:"Clear Errors.vi"("error in (no error)"=w375) -> ()  [unwired: 6 in, 1 out]
              }
            }
          }
          event #4 {
            n192 = event-data() -> ()  [unwired: 1 in, 5 out]
            n193 = local read "Config Rigol DP832"() -> (w415:T13)
            n194 = local read "VISA Rigol DP832"() -> (w414:refnum<visa-resource-name>)
            n195 = case shown="True" "CHECK cta" {
              tunnel: w414 -> [w419 w451]
              tunnel: w415 -> [w418 w450]
              frame #0 {
                w417 = errorcluster {"status"=FALSE, "code"=0, "source"=""} ("error in")
                n196 = call "DP832_Enable ALL Output.vi"("Enable Output (T: Enable)"=FALSE, "error in (no error)"=w417, "VISA resource name"=w419) -> ("error out"=w424:errorcluster, "VISA resource name out"=w425:refnum<visa-resource-name>)  [unwired: 7 in]
                n197 = for {
                  shift-right: [w434] -> w420
                  shift-left: w424 -> [w430]
                  shift-right: [w435] -> w421
                  shift-left: w425 -> [w431]
                  tunnel: w418 -> [w429] mode=indexing
                  w428 = 0.0  # Voltage Level
                  w432 = 0.0  # Current Limit
                  w436 = T22 0 items=["Regulate", "Trip"] ("Behavior (0: Regulate)")
                  n198 = Unbundle By Name(w429) -> ("Channel"=w433:T3)
                  n199 = call "DP832_Configure Current Limit.vi"("Behavior"=w436, "error in (no error)"=w430, "Current Limit"=w432, "Channel"=w433, "VISA resource name"=w431) -> ("error out"=w438:errorcluster, "VISA resource name out"=w439:refnum<visa-resource-name>)  [unwired: 5 in]
                  n200 = call "DP832_Configure Output.vi"("Enable Output (T: Enable)"=FALSE, "error in (no error)"=w438, "Voltage Level"=w428, "Channel"=w433, "VISA resource name"=w439) -> ("error out"=w434:errorcluster, "VISA resource name out"=w435:refnum<visa-resource-name>)  [unwired: 5 in]
                }
                n201 = flat-sequence {
                  tunnel: w417 -> [_]
                  frame #0 {
                    n202 = local read "FT_Handle"() -> (w427:u32)
                    n203 = call "FT_Close_Device.vi"("Handle"=w427) -> ()  [unwired: 1 out]
                  }
                }
                n204 = call "DP832_Local Mode.vi"("error in (no error)"=w420, "VISA resource name"=w421) -> ("error out"=w423:errorcluster, "VISA resource name out"=w422:refnum<visa-resource-name>)  [unwired: 8 in]
                n205 = call "DP832_Close.vi"("error in (no error)"=w423, "VISA resource name"=w422) -> ("error out"=w416:errorcluster)  [unwired: 8 in, 1 out]
                n206 = call <vilib>:"Clear Errors.vi"("error in (no error)"=w416) -> ()  [unwired: 6 in, 1 out]
              }
              frame #1 {
                n207 = property on="CTA Board" class="CmbBox"() -> ("Value"=w445:string)  [unwired: 2 in, 2 out]
                n208 = for {
                  N: 3 -> [_]
                  tunnel: [w460] -> w449
                  tunnel: w450 -> [w466]
                  tunnel: w451 -> [w463]
                  tunnel: errorcluster {"status"=FALSE, "code"=0, "source"=""} ("error in") -> [w462]
                  stop <- w458 continue-if-true
                  n209 = call "Prueba_rigol.vi"("error in (no error)"=w462, "VISA IN"=w463) -> ("error out 2"=w461:errorcluster)  [unwired: 8 in, 1 out]
                  n210 = call "DP832_Init gustavo.vi"("error in (no error)"=w461, "VISA resource name 2"=w463) -> ("error out"=w464:errorcluster, "VISA resource name"=w465:refnum<visa-resource-name>)
                  n211 = call "DP832_Beep.vi"("error in (no error)"=w464, "VISA resource name"=w465) -> ("error out"=w470:errorcluster, "VISA resource name out"=w471:refnum<visa-resource-name>)  [unwired: 8 in]
                  n212 = for {
                    shift-right: [w477] -> w468
                    shift-left: w470 -> [w479]
                    shift-right: [w478] -> w469
                    shift-left: w471 -> [w480]
                    tunnel: w466 -> [w476] mode=indexing
                    w481 = T22 0 items=["Regulate", "Trip"] ("Behavior (0: Regulate)")
                    n213 = Unbundle By Name(w476) -> ("Channel"=w474:T3, "V Limit"=w475:dbl, "I Limit"=w473:dbl, "V Out"=w472:dbl)
                    n214 = call "DP832_Configure OVP.vi"("Enable OVP (T: Enable)"=FALSE, "error in (no error)"=w479, "Voltage Limit"=w475, "Channel"=w474, "VISA resource name"=w480) -> ("error out"=w484:errorcluster, "VISA resource name out"=w483:refnum<visa-resource-name>)  [unwired: 5 in]
                    n215 = call "DP832_Configure Current Limit.vi"("Behavior"=w481, "error in (no error)"=w484, "Current Limit"=w473, "Channel"=w474, "VISA resource name"=w483) -> ("error out"=w486:errorcluster, "VISA resource name out"=w487:refnum<visa-resource-name>)  [unwired: 5 in]
                    n216 = call "DP832_Configure Output.vi"("Enable Output (T: Enable)"=FALSE, "error in (no error)"=w486, "Voltage Level"=w472, "Channel"=w474, "VISA resource name"=w487) -> ("error out"=w477:errorcluster, "VISA resource name out"=w478:refnum<visa-resource-name>)  [unwired: 5 in]
                  }
                  n217 = call "DP832_Enable ALL Output.vi"("Enable Output (T: Enable)"=TRUE, "error in (no error)"=w468, "VISA resource name"=w469) -> ("error out"=w460:errorcluster)  [unwired: 7 in, 1 out]
                  n218 = Select(t=TRUE, s=w460, f=FALSE) -> (s? t:f=w458:bool)
                }
                n219 = call <vilib>:"Clear Errors.vi"("error in (no error)"=w449) -> ("error out"=w441:errorcluster)  [unwired: 6 in]
                n220 = call "FT_Search All Select description.vi"("error in (no error)"=w441, "CTA Test#"=w445) -> ("error Out"=w440:errorcluster, "All FT"=w446:T23, "Select Ft"=w448:T24)  [unwired: 7 in]
                n221 = call <vilib>:"Clear Errors.vi"("error in (no error)"=w440) -> ()  [unwired: 6 in, 1 out]
                n222 = for {
                  tunnel: w446 -> [w456] mode=indexing
                  tunnel: [w454] -> w444 mode=indexing
                  n223 = Unbundle By Name(w456) -> ("Serial Number"=w455:string)
                  n224 = Bundle("Serial Number"=w455, "Serial Number"=w455) -> (w454:T25)  [unwired: 1 in]
                }
                n225 = Unbundle By Name(w448) -> ("FT_Handle"=→"FT_Handle":u32)
                n226 = property on="CTA Board" class="CmbBox"("Strings And Values[]"=w444) -> (error out=w442:errorcluster)  [unwired: 2 in, 1 out]
                n227 = property on="CHECK cta" class="Bool (strict)"(error in=w442, "Val(Sgnl)"=FALSE) -> ()  [unwired: 1 in, 2 out]
              }
            }
          }
          event #5 {
            n228 = event-data() -> ()  [unwired: 1 in, 5 out]
            n229 = local read "Config Rigol DP832"() -> (w493:T13)
            n230 = local read "VISA Rigol DP832"() -> (w492:refnum<visa-resource-name>)
            n231 = case shown="True" "CHECK vga" {
              tunnel: w492 -> [w496 w528]
              tunnel: w493 -> [w495 w523]
              frame #0 {
                w494 = errorcluster {"status"=FALSE, "code"=0, "source"=""} ("error in")
                n232 = call "DP832_Enable ALL Output.vi"("Enable Output (T: Enable)"=FALSE, "error in (no error)"=w494, "VISA resource name"=w496) -> ("error out"=w501:errorcluster, "VISA resource name out"=w502:refnum<visa-resource-name>)  [unwired: 7 in]
                n233 = flat-sequence {
                  tunnel: w494 -> [_]
                  frame #0 {
                    n234 = property on="VGA" class="Clust (strict)"("Visible"=TRUE) -> ()  [unwired: 2 in, 2 out]
                    n235 = local read "FT_Handle"() -> (w507:u32)
                    n236 = property on="QUIT" class="Bool"("DisabledEnum"=T17."Enabled" ("Disabled")) -> ()  [unwired: 2 in, 2 out]
                    n237 = call "FT_Close_Device.vi"("Handle"=w507) -> ()  [unwired: 1 out]
                    n238 = property on="vga test" class="Clust (strict)"("Visible"=FALSE) -> ()  [unwired: 2 in, 2 out]
                  }
                }
                n239 = for {
                  shift-right: [w514] -> w497
                  shift-left: w501 -> [w510]
                  shift-right: [w515] -> w498
                  shift-left: w502 -> [w511]
                  tunnel: w495 -> [w509] mode=indexing
                  w508 = 0.0  # Voltage Level
                  w512 = 0.0  # Current Limit
                  w516 = T22 0 items=["Regulate", "Trip"] ("Behavior (0: Regulate)")
                  n240 = Unbundle By Name(w509) -> ("Channel"=w513:T3)
                  n241 = call "DP832_Configure Current Limit.vi"("Behavior"=w516, "error in (no error)"=w510, "Current Limit"=w512, "Channel"=w513, "VISA resource name"=w511) -> ("error out"=w518:errorcluster, "VISA resource name out"=w519:refnum<visa-resource-name>)  [unwired: 5 in]
                  n242 = call "DP832_Configure Output.vi"("Enable Output (T: Enable)"=FALSE, "error in (no error)"=w518, "Voltage Level"=w508, "Channel"=w513, "VISA resource name"=w519) -> ("error out"=w514:errorcluster, "VISA resource name out"=w515:refnum<visa-resource-name>)  [unwired: 5 in]
                }
                n243 = call "DP832_Local Mode.vi"("error in (no error)"=w497, "VISA resource name"=w498) -> ("error out"=w500:errorcluster, "VISA resource name out"=w499:refnum<visa-resource-name>)  [unwired: 8 in]
                n244 = call "DP832_Close.vi"("error in (no error)"=w500, "VISA resource name"=w499) -> ()  [unwired: 8 in, 2 out]
              }
              frame #1 {
                w520 = errorcluster {"status"=FALSE, "code"=0, "source"=""} ("error in")
                n245 = property on="CTA Board" class="CmbBox"() -> ("Value"=w525:string)  [unwired: 2 in, 2 out]
                n246 = for {
                  N: 3 -> [_]
                  tunnel: [w541] -> w527
                  tunnel: w523 -> [w547]
                  tunnel: w528 -> [w544]
                  tunnel: w520 -> [w543]
                  stop <- w539 continue-if-true
                  n247 = call "Prueba_rigol.vi"("error in (no error)"=w543, "VISA IN"=w544) -> ("error out 2"=w542:errorcluster)  [unwired: 8 in, 1 out]
                  n248 = call "DP832_Init gustavo.vi"("error in (no error)"=w542, "VISA resource name 2"=w544) -> ("error out"=w545:errorcluster, "VISA resource name"=w546:refnum<visa-resource-name>)
                  n249 = call "DP832_Beep.vi"("error in (no error)"=w545, "VISA resource name"=w546) -> ("error out"=w551:errorcluster, "VISA resource name out"=w552:refnum<visa-resource-name>)  [unwired: 8 in]
                  n250 = for {
                    shift-right: [w558] -> w549
                    shift-left: w551 -> [w560]
                    shift-right: [w559] -> w550
                    shift-left: w552 -> [w561]
                    tunnel: w547 -> [w557] mode=indexing
                    w562 = T22 0 items=["Regulate", "Trip"] ("Behavior (0: Regulate)")
                    n251 = Unbundle By Name(w557) -> ("Channel"=w555:T3, "V Limit"=w556:dbl, "I Limit"=w554:dbl, "V Out"=w553:dbl)
                    n252 = call "DP832_Configure OVP.vi"("Enable OVP (T: Enable)"=FALSE, "error in (no error)"=w560, "Voltage Limit"=w556, "Channel"=w555, "VISA resource name"=w561) -> ("error out"=w565:errorcluster, "VISA resource name out"=w564:refnum<visa-resource-name>)  [unwired: 5 in]
                    n253 = call "DP832_Configure Current Limit.vi"("Behavior"=w562, "error in (no error)"=w565, "Current Limit"=w554, "Channel"=w555, "VISA resource name"=w564) -> ("error out"=w567:errorcluster, "VISA resource name out"=w568:refnum<visa-resource-name>)  [unwired: 5 in]
                    n254 = call "DP832_Configure Output.vi"("Enable Output (T: Enable)"=FALSE, "error in (no error)"=w567, "Voltage Level"=w553, "Channel"=w555, "VISA resource name"=w568) -> ("error out"=w558:errorcluster, "VISA resource name out"=w559:refnum<visa-resource-name>)  [unwired: 5 in]
                  }
                  n255 = call "DP832_Enable ALL Output.vi"("Enable Output (T: Enable)"=TRUE, "error in (no error)"=w549, "VISA resource name"=w550) -> ("error out"=w541:errorcluster)  [unwired: 7 in, 1 out]
                  n256 = Select(t=TRUE, s=w541, f=FALSE) -> (s? t:f=w539:bool)
                }
                n257 = property on="QUIT" class="Bool"(error in=w520, "DisabledEnum"=T17."Disabled and Grayed Out" ("Disabled")) -> ()  [unwired: 1 in, 2 out]
                n258 = flat-sequence {
                  tunnel: w524 -> [_]
                  frame #0 {
                    n259 = local read "VGA"() -> (w535:T14)
                    n260 = Unbundle By Name(w535) -> ("TIME VGA.PULSE WIDTH"=w532:u16, "TIME VGA.FRECUENCY PULSE"=w531:dbl)
                    n261 = property on="vga test" class="Clust (strict)"("Visible"=TRUE) -> ()  [unwired: 2 in, 2 out]
                    n262 = property on="VGA" class="Clust (strict)"("Visible"=FALSE) -> ()  [unwired: 2 in, 2 out]
                    n263 = Bundle By Name(cluster=T12 {"FRECUENCY PULSE"=0.0, "PULSE WIDTH"=0, "CODE GAIN TEST"=0} ("Value (Signaling)"), "CODE GAIN TEST"=u8 0, "PULSE WIDTH"=w532, "FRECUENCY PULSE"=w531) -> (w533:T12)
                    n264 = property on="vga test" class="Clust (strict)"("Val(Sgnl)"=w533) -> ()  [unwired: 2 in, 2 out]
                  }
                }
                n265 = call <vilib>:"Clear Errors.vi"("error in (no error)"=w527) -> ("error out"=w522:errorcluster)  [unwired: 6 in]
                n266 = call "FT_Search All Select description.vi"("error in (no error)"=w522, "CTA Test#"=w525) -> ("Select Ft"=w526:T24)  [unwired: 7 in, 2 out]
                n267 = Unbundle By Name(w526) -> ("FT_Handle"=w524:u32)
                n268 = local write "FT_Handle"(w524) -> ()
              }
            }
          }
          event #6 {
            w576 = u32 20 ("Espera acceso USB")
            n269 = event-data() -> ()  [unwired: 1 in, 5 out]
            n270 = Unbundle By Name("vga test") -> ("PULSE WIDTH"=w573:u16, "FRECUENCY PULSE"=w571:dbl, "CODE GAIN TEST"=w572:u8)
            n271 = local read "FT_Handle"() -> (w577:u32)
            n272 = call "VGA_pulso.vi"("Espera acceso USB"=w576, "Frecuencia pulso (0.2 a 1 Mhz)"=w571, "Patrón (E000)"=w573, "ftHandle_in"=w577) -> ("error out"=w578:errorcluster, "ftHandle_out"=w579:u32)  [unwired: 6 in]
            n273 = call "VGA_ganancia.vi"("Espera acceso USB"=w576, "error in 2"=w578, "Ganancia"=w572, "ftHandle_in 2"=w579) -> ()  [unwired: 6 in, 2 out]
          }
          event #7 {
            n274 = event-data() -> ("NewVal"=w594:i32)  [unwired: 1 in, 4 out]
            n275 = property on="Valores" class="Arr (strict)"() -> ("Value"=w581:T15[])  [unwired: 2 in, 2 out]
            n276 = Array Size(array=w581) -> (size(s)=w598:i32)
            n277 = Decrement(x=w598) -> (x-1=w588:i32)
            n278 = Less Than 0?(x=w588) -> (x < 0?=w590:bool)
            n279 = Select(t=0 ("x"), s=w590, f=w588) -> (s? t:f=w587:i32)
            n280 = In Range and Coerce(upper limit=w587, x=w594, lower limit=0 ("x")) -> (coerced(x)=w595:i32, In Range?=w596:bool)
            n281 = for {
              tunnel: [w601] -> w583 mode=indexing
              tunnel: w581 -> [w600] mode=indexing
              n282 = Unbundle By Name(w600) -> ("VOLTAGE SUPPLY ASIC"=w601:dbl)
            }
            n283 = Select(t=w594, s=w596, f=w595) -> (s? t:f=w580:i32)
            n284 = property on="TEST#" class="DigNum (strict)"("Value"=w580) -> (error out=w592:errorcluster)  [unwired: 2 in, 1 out]
            n285 = Build Array(w580) -> (w593:i32[])
            n286 = property on="Valores" class="Arr (strict)"(error in=w592, "Index Values"=w593) -> ()  [unwired: 1 in, 2 out]
            n287 = Number To Fractional String(number=w583, width (-)=i16 1, precision (6)=i16 2) -> (F-format string=w582:string[])  [unwired: 1 in]
            n288 = property on="Elemensts" class="LstBox (strict)"("EditRow"=w580, "Item Names"=w582) -> ()  [unwired: 2 in, 2 out]
          }
          event #8 {
            n289 = event-data() -> ()  [unwired: 1 in, 5 out]
            n290 = property on="Valores" class="Arr (strict)"() -> ("Index Values"=w607:u32[], "Value"=w606:T15[])  [unwired: 2 in, 2 out]
            n291 = for {
              tunnel: [w611] -> w603 mode=indexing
              tunnel: w606 -> [w610] mode=indexing
              n292 = Unbundle By Name(w610) -> ("VOLTAGE SUPPLY ASIC"=w611:dbl)
            }
            n293 = Index Array(array=w607, index=0) -> (element=w609:u32)
            n294 = Number To Fractional String(number=w603, width (-)=i16 1, precision (6)=i16 2) -> (F-format string=w602:string[])  [unwired: 1 in]
            n295 = property on="Elemensts" class="LstBox (strict)"("EditRow"=w609, "Item Names"=w602) -> ()  [unwired: 2 in, 2 out]
          }
          event #9 {
            n296 = event-data() -> ()  [unwired: 1 in, 5 out]
            n297 = call "gui.default values test.vi"() -> ("Values default"=w631:T21)  [unwired: 8 in, 3 out]
            n298 = property on="Valores" class="Arr (strict)"() -> ("Value"=w626:T15[])  [unwired: 2 in, 2 out]
            n299 = Index Array(array=w631, index=1) -> (element=w630:T26)
            n300 = Unbundle By Name(w630) -> ("Vsupply asic"=w681:dbl, "Test Register??"=w619:bool, "Test ADC??"=w680:bool, "Test ADC set.Repeats ADC"=w679:i32, "Test ADC set.Max Desviation"=w678:dbl, "High ADC means"=w675:dbl[], "Low ADC means"=w674:dbl[], "Test MAX/MIN??"=w671:bool, "Limits Max PN Min NP.Max P Lower"=w670:dbl, "Limits Max PN Min NP.Min P Lower"=w669:dbl, "Limits Max PN Min NP.Max N Lower"=w668:dbl, "Limits Max PN Min NP.Min N Lower"=w667:dbl, "Limits Max PN Min NP.Max P Upper"=w635:dbl, "Limits Max PN Min NP.Min P Upper"=w634:dbl, "Limits Max PN Min NP.Max N Upper"=w633:dbl, "Limits Max PN Min NP.Min N Upper"=w632:dbl, "Test rate scan"=w660:bool, "Vin Rate Scan"=w659:i32[], "High rate scan"=w638:dbl[], "Low rate scan"=w639:dbl[], "Test rate scan adders??"=w654:bool, "Vin Rate Adders"=w653:i32[], "High rate scan add"=w636:dbl[], "Low rate scan add"=w637:dbl[], "Test offset analog??"=w648:bool, "Lim Offset Analog.Max Analog"=w647:dbl, "Lim Offset Analog.Min Analog"=w646:dbl, "Test offset digital??"=w645:bool, "Lim offset Dig.Max Dig"=w644:dbl)
            n301 = Build Array(w637, w636) -> (w652:dbl[][])
            n302 = Build Array(w635, w634, w633, w632) -> (w665:dbl[])
            n303 = Build Array(w639, w638) -> (w656:dbl[][])
            n304 = Build Array(w674, w675) -> (w673:dbl[][])
            n305 = Build Array(w670, w669, w668, w667) -> (w666:dbl[])
            n306 = Transpose 2D Array(2D array=w656) -> (transposed array=w641:dbl[][])
            n307 = Transpose 2D Array(2D array=w673) -> (transposed array=w643:dbl[][])
            n308 = Transpose 2D Array(2D array=w652) -> (transposed array=w640:dbl[][])
            n309 = Build Array(w666, w665) -> (w662:dbl[][])
            n310 = Transpose 2D Array(2D array=w662) -> (transposed array=w642:dbl[][])
            n311 = Number To Fractional String(number=w641, width (-)=i16 1, precision (6)=i16 4) -> (F-format string=w655:string[][])  [unwired: 1 in]
            n312 = Number To Fractional String(number=w643, width (-)=i16 1, precision (6)=i16 4) -> (F-format string=w672:string[][])  [unwired: 1 in]
            n313 = Number To Fractional String(number=w640, width (-)=i16 1, precision (6)=i16 4) -> (F-format string=w649:string[][])  [unwired: 1 in]
            n314 = Number To Fractional String(number=w642, width (-)=i16 1, precision (6)=i16 4) -> (F-format string=w661:string[][])  [unwired: 1 in]
            n315 = Index Array(array=w626, index=0) -> (element=w682:T15)
            n316 = Bundle By Name(cluster=w682, "VOLTAGE SUPPLY ASIC"=w681, "TEST REGISTER"=w619, "TEST ADC"=w680, "SETUP ADC 2.NUMBER OF REPETITIONS"=w679, "SETUP ADC 2.MAX DESVIATION ADC"=w678, "LIMITS MEASUREMENT ADC"=w672, "TEST MAX MIN P/N"=w671, "LIMITS MAX PN MIN NP"=w661, "TEST RATE SCAN"=w660, "VIN ASIC"=w659, "LIMITS RATE SCAN"=w655, "TEST RATE SCAN ADDERS"=w654, "VIN ASIC ADD"=w653, "LIMITS RATE SCAN ADDERS"=w649, "TEST OFFSET ANALOG"=w648, "LIMITS OFFSET ANALOG.MAXIMUM"=w647, "LIMITS OFFSET ANALOG.MINIMUM"=w646, "TEST OFFSET DIGITAL"=w645, "LIMITS OFFSET DIGITAL.MAXIMUM"=w644) -> (w625:T15)
            n317 = Build Array (concatenate)(w626, w625) -> (w614:T15[])
            n318 = Array Size(array=w614) -> (size(s)=w622:i32)
            n319 = property on="Valores" class="Arr (strict)"("Value"=w614) -> (error out=w624:errorcluster)  [unwired: 2 in, 1 out]
            n320 = Decrement(x=w622) -> (x-1=w612:i32)
            n321 = property on="Valores" class="Arr (strict)"(error in=w624, "Val(Sgnl)"=w614) -> ()  [unwired: 1 in, 2 out]
            n322 = for {
              tunnel: [w684] -> w613 mode=indexing
              tunnel: w614 -> [w683] mode=indexing
              n323 = Unbundle By Name(w683) -> ("VOLTAGE SUPPLY ASIC"=w684:dbl)
            }
            n324 = Build Array(w612) -> (w621:i32[])
            n325 = Number To Fractional String(number=w613, width (-)=i16 1, precision (6)=i16 2) -> (F-format string=w615:string[])  [unwired: 1 in]
            n326 = property on="Valores" class="Arr (strict)"("Index Values"=w621) -> (error out=w620:errorcluster)  [unwired: 2 in, 1 out]
            n327 = property on="TEST#" class="DigNum (strict)"(error in=w620, "Value"=w612) -> ()  [unwired: 1 in, 2 out]
            n328 = property on="Elemensts" class="LstBox (strict)"("EditRow"=w612, "Item Names"=w615) -> ()  [unwired: 2 in, 2 out]
          }
          event #10 {
            n329 = event-data() -> ()  [unwired: 1 in, 5 out]
          }
          event #11 {
            n330 = event-data() -> ()  [unwired: 1 in, 5 out]
            n331 = property on="Valores" class="Arr (strict)"() -> ("Value"=w694:T15[], "Index Values"=w701:u32[])  [unwired: 2 in, 2 out]
            n332 = Index Array(array=w701, index=0) -> (element=w699:u32)
            n333 = Index Array(array=w694, index=w699) -> (element=w706:T15)
            n334 = Build Array (concatenate)(w694, w706) -> (w689:T15[])
            n335 = property on="Valores" class="Arr (strict)"("Value"=w689) -> (error out=w697:errorcluster)  [unwired: 2 in, 1 out]
            n336 = property on="Valores" class="Arr (strict)"(error in=w697, "Val(Sgnl)"=w689) -> (error out=w705:errorcluster)  [unwired: 1 in, 1 out]
            n337 = Array Size(array=w689) -> (size(s)=w698:i32)
            n338 = for {
              tunnel: [w708] -> w690 mode=indexing
              tunnel: w689 -> [w707] mode=indexing
              n339 = Unbundle By Name(w707) -> ("VOLTAGE SUPPLY ASIC"=w708:dbl)
            }
            n340 = Decrement(x=w698) -> (x-1=w688:i32)
            n341 = Build Array(w688) -> (w703:i32[])
            n342 = property on="Valores" class="Arr (strict)"(error in=w705, "Index Values"=w703) -> (error out=w704:errorcluster)  [unwired: 1 in, 1 out]
            n343 = property on="TEST#" class="DigNum (strict)"(error in=w704, "Value"=w688) -> ()  [unwired: 1 in, 2 out]
            n344 = Number To Fractional String(number=w690, width (-)=i16 1, precision (6)=i16 2) -> (F-format string=w691:string[])  [unwired: 1 in]
            n345 = property on="Elemensts" class="LstBox (strict)"("EditRow"=w688, "Item Names"=w691) -> ()  [unwired: 2 in, 2 out]
          }
          event #12 {
            n346 = event-data() -> ()  [unwired: 1 in, 5 out]
            n347 = property on="Valores" class="Arr (strict)"() -> ("Value"=w716:T15[])  [unwired: 2 in, 2 out]
            n348 = Array Size(array=w716) -> (size(s)=w715:i32)
            n349 = Decrement(x=w715) -> (x-1=w711:i32)
            n350 = Greater Or Equal?(x=w711, y=0) -> (x >= y?=w713:bool)
            n351 = case shown="True" w713 {
              frame #0 {
              }
              frame #1 {
                n352 = property on="Valores" class="Arr (strict)"() -> ("Value"=w723:T15[], "Index Values"=w725:u32[])  [unwired: 2 in, 2 out]
                n353 = Index Array(array=w725, index=0) -> (element=w717:u32)
                n354 = Delete From Array(array=w723, length=1, index=w717) -> (array with subset deleted=w718:T15[])  [unwired: 1 out]
                n355 = for {
                  tunnel: w718 -> [w731] mode=indexing
                  tunnel: [w730] -> w720 mode=indexing
                  n356 = Unbundle By Name(w731) -> ("VOLTAGE SUPPLY ASIC"=w730:dbl)
                }
                n357 = property on="Valores" class="Arr (strict)"("Val(Sgnl)"=w718) -> (error out=w727:errorcluster)  [unwired: 2 in, 1 out]
                n358 = property on="Valores" class="Arr (strict)"(error in=w727, "Index Values"=u32[] [0]) -> (error out=w726:errorcluster)  [unwired: 1 in, 1 out]
                n359 = Number To Fractional String(number=w720, width (-)=i16 1, precision (6)=i16 2) -> (F-format string=w719:string[])  [unwired: 1 in]
                n360 = property on="Elemensts" class="LstBox (strict)"("EditRow"=w717, "Item Names"=w719) -> ()  [unwired: 2 in, 2 out]
                n361 = property on="TEST#" class="DigNum (strict)"(error in=w726, "Val(Sgnl)"=w717) -> ()  [unwired: 1 in, 2 out]
              }
            }
          }
          event #13 {
            n362 = event-data() -> ()  [unwired: 1 in, 5 out]
          }
          event #14 {
            n363 = event-data() -> ()  [unwired: 1 in, 5 out]
            n364 = Unbundle By Name(w755) -> ("Config Test"=w758:T4)
            n365 = Index Array(array=w758, index=0) -> (element=w756:T5)
            n366 = for {
              tunnel: "Valores" -> [w812] mode=indexing
              tunnel: w756 -> [w811]
              tunnel: [w795] -> w737 mode=indexing
              n367 = Unbundle By Name(w812) -> ("VOLTAGE SUPPLY ASIC"=w810:dbl, "TEST REGISTER"=w768:bool, "TEST ADC"=w809:bool, "SETUP ADC 2.NUMBER OF REPETITIONS"=w808:i32, "SETUP ADC 2.MAX DESVIATION ADC"=w807:dbl, "LIMITS MEASUREMENT ADC"=w799:string[][], "TEST MAX MIN P/N"=w806:bool, "LIMITS MAX PN MIN NP"=w794:string[][], "TEST RATE SCAN"=w805:bool, "VIN ASIC"=w804:i32[], "LIMITS RATE SCAN"=w789:string[][], "TEST RATE SCAN ADDERS"=w803:bool, "VIN ASIC ADD"=w802:i32[], "LIMITS RATE SCAN ADDERS"=w763:string[][], "TEST OFFSET ANALOG"=w767:bool, "LIMITS OFFSET ANALOG.MAXIMUM"=w785:dbl, "LIMITS OFFSET ANALOG.MINIMUM"=w784:dbl, "TEST OFFSET DIGITAL"=w801:bool, "LIMITS OFFSET DIGITAL.MAXIMUM"=w800:dbl)
              n368 = Fract/Exp String To Number(string=w794) -> (number=w771:dbl[][])  [unwired: 3 in, 1 out]
              n369 = Fract/Exp String To Number(string=w763) -> (number=w764:dbl[][])  [unwired: 3 in, 1 out]
              n370 = Fract/Exp String To Number(string=w799) -> (number=w798:dbl[][])  [unwired: 3 in, 1 out]
              n371 = Fract/Exp String To Number(string=w789) -> (number=w788:dbl[][])  [unwired: 3 in, 1 out]
              n372 = Index Array(array=w771, index (col) #1=0 ("index (row)"), index (col) #2=1 ("index (row)")) -> (element #1=w793:dbl[], element #2=w791:dbl[])  [unwired: 2 in]
              n373 = Index Array(array=w764, index (col) #1=1 ("index (row)"), index (col) #2=0 ("index (row)")) -> (element #1=w762:dbl[], element #2=w761:dbl[])  [unwired: 2 in]
              n374 = Index Array(array=w798, index (col) #1=0 ("index (row)"), index (col) #2=1 ("index (row)")) -> (element #1=w797:dbl[], element #2=w796:dbl[])  [unwired: 2 in]
              n375 = Index Array(array=w793, index #1=0 ("index")) -> (element #1=w781:dbl, element #2=w780:dbl, element #3=w779:dbl, element #4=w778:dbl)  [unwired: 3 in]
              n376 = Index Array(array=w791, index #1=0 ("index")) -> (element #1=w777:dbl, element #2=w776:dbl, element #3=w775:dbl, element #4=w774:dbl)  [unwired: 3 in]
              n377 = Index Array(array=w788, index (col) #1=1 ("index (row)"), index (col) #2=0 ("index (row)")) -> (element #1=w787:dbl[], element #2=w786:dbl[])  [unwired: 2 in]
              n378 = Bundle By Name(cluster=w811, "Vasic"=w810, "Test Register?"=w768, "Test ADC?"=w809, "Test ADC.Repeats ADC"=w808, "Test ADC.Max Desviation"=w807, "Limits ADC.Low"=w797, "Limits ADC.High"=w796, "Test Max PN Min NP?"=w806, "Limits Max PN Min NP.Max P Lower"=w781, "Limits Max PN Min NP.Min P Lower"=w780, "Limits Max PN Min NP.Max N Lower"=w779, "Limits Max PN Min NP.Min N Lower"=w778, "Limits Max PN Min NP.Max P Upper"=w777, "Limits Max PN Min NP.Min P Upper"=w776, "Limits Max PN Min NP.Max N Upper"=w775, "Limits Max PN Min NP.Min N Upper"=w774, "Test Rate Scan?"=w805, "Vin Rate Scan"=w804, "Limits Rate Scan.High"=w787, "Limits Rate Scan.Low"=w786, "Test Rate Scan Adders?"=w803, "Vin Rate Adders"=w802, "Limits Rate Scan adders.High"=w762, "Limits Rate Scan adders.Low"=w761, "Test offset analog?"=w767, "Lim Offset Analog.Max Analog"=w785, "Lim Offset Analog.Min Analog"=w784, "Test offset digital?"=w801, "Lim offset Dig.Max Dig"=w800) -> (w795:T5)
            }
            n379 = property on="CTA Board" class="CmbBox"() -> ("Value"=w735:string)  [unwired: 2 in, 2 out]
            n380 = Unbundle By Name("VGA") -> ("VALUES VGA"=w750:string[][], "TIME VGA.PULSE WIDTH"=w751:u16, "TIME VGA.FRECUENCY PULSE"=w752:dbl)
            n381 = property on="VALUES VGA" class="Tbl (strict)"() -> ("Row Headers[]"=w745:string[])  [unwired: 2 in, 2 out]
            n382 = Fract/Exp String To Number(string=w745) -> (number=w740:dbl[])  [unwired: 3 in, 1 out]
            n383 = Divide(x=w740, y=1000.0) -> (x/y=w741:dbl[])
            n384 = Index Array(array=w750, index (col) #1=1 ("disabled index (col)"), index (col) #2=0 ("index (col)")) -> (element #1=w747:string[], element #2=w749:string[])  [unwired: 2 in]
            n385 = Fract/Exp String To Number(string=w747) -> (number=w746:dbl[])  [unwired: 3 in, 1 out]
            n386 = Decimal String To Number(string=w749) -> (number=w748:i32[])  [unwired: 2 in, 1 out]
            n387 = Bundle By Name(cluster=w755, "Config HW.Config Rigol DP832"="Config Rigol DP832", "Config HW.VISA Rigol DP832"="VISA Rigol DP832", "Config HW.CTA Test#"=w735, "Config VGA.Theoretical Voltage"=w741, "Config VGA.Real Voltage"=w746, "Config VGA.VGA Gain"=w748, "Config VGA.Pulse Width"=w751, "Config VGA.Frecuency Pulse"=w752, "Config Test"=w737) -> (w738:T1)
          }
        }
      }
      frame #9 {
        n388 = Unbundle By Name(w822) -> ("Config Test"=w823:T4)
        n389 = local read "Valores"() -> (w818:T15[])
        n390 = Index Array(array=w823, index=0) -> (element=w825:T5)
        n391 = for {
          tunnel: w818 -> [w890] mode=indexing
          tunnel: w825 -> [w889]
          tunnel: [w872] -> w838 mode=indexing
          n392 = Unbundle By Name(w890) -> ("VOLTAGE SUPPLY ASIC"=w888:dbl, "TEST REGISTER"=w845:bool, "TEST ADC"=w887:bool, "SETUP ADC 2.NUMBER OF REPETITIONS"=w886:i32, "SETUP ADC 2.MAX DESVIATION ADC"=w885:dbl, "LIMITS MEASUREMENT ADC"=w876:string[][], "TEST MAX MIN P/N"=w884:bool, "LIMITS MAX PN MIN NP"=w871:string[][], "TEST RATE SCAN"=w883:bool, "VIN ASIC"=w882:i32[], "LIMITS RATE SCAN"=w866:string[][], "TEST RATE SCAN ADDERS"=w881:bool, "VIN ASIC ADD"=w880:i32[], "LIMITS RATE SCAN ADDERS"=w841:string[][], "TEST OFFSET ANALOG"=w879:bool, "LIMITS OFFSET ANALOG.MAXIMUM"=w862:dbl, "LIMITS OFFSET ANALOG.MINIMUM"=w861:dbl, "TEST OFFSET DIGITAL"=w878:bool, "LIMITS OFFSET DIGITAL.MAXIMUM"=w877:dbl)
          n393 = Fract/Exp String To Number(string=w841) -> (number=w842:dbl[][])  [unwired: 3 in, 1 out]
          n394 = Fract/Exp String To Number(string=w866) -> (number=w865:dbl[][])  [unwired: 3 in, 1 out]
          n395 = Fract/Exp String To Number(string=w871) -> (number=w848:dbl[][])  [unwired: 3 in, 1 out]
          n396 = Index Array(array=w865, index (col) #1=1 ("index (row)"), index (col) #2=0 ("index (row)")) -> (element #1=w864:dbl[], element #2=w863:dbl[])  [unwired: 2 in]
          n397 = Fract/Exp String To Number(string=w876) -> (number=w875:dbl[][])  [unwired: 3 in, 1 out]
          n398 = Index Array(array=w842, index (col) #1=1 ("index (row)"), index (col) #2=0 ("index (row)")) -> (element #1=w840:dbl[], element #2=w839:dbl[])  [unwired: 2 in]
          n399 = Index Array(array=w848, index (col) #1=0 ("index (row)"), index (col) #2=1 ("index (row)")) -> (element #1=w870:dbl[], element #2=w868:dbl[])  [unwired: 2 in]
          n400 = Index Array(array=w875, index (col) #1=0 ("index (row)"), index (col) #2=1 ("index (row)")) -> (element #1=w874:dbl[], element #2=w873:dbl[])  [unwired: 2 in]
          n401 = Index Array(array=w870, index #1=0 ("index")) -> (element #1=w858:dbl, element #2=w857:dbl, element #3=w856:dbl, element #4=w855:dbl)  [unwired: 3 in]
          n402 = Index Array(array=w868, index #1=0 ("index")) -> (element #1=w854:dbl, element #2=w853:dbl, element #3=w852:dbl, element #4=w851:dbl)  [unwired: 3 in]
          n403 = Bundle By Name(cluster=w889, "Vasic"=w888, "Test Register?"=w845, "Test ADC?"=w887, "Test ADC.Repeats ADC"=w886, "Test ADC.Max Desviation"=w885, "Limits ADC.Low"=w874, "Limits ADC.High"=w873, "Test Max PN Min NP?"=w884, "Limits Max PN Min NP.Max P Lower"=w858, "Limits Max PN Min NP.Min P Lower"=w857, "Limits Max PN Min NP.Max N Lower"=w856, "Limits Max PN Min NP.Min N Lower"=w855, "Limits Max PN Min NP.Max P Upper"=w854, "Limits Max PN Min NP.Min P Upper"=w853, "Limits Max PN Min NP.Max N Upper"=w852, "Limits Max PN Min NP.Min N Upper"=w851, "Test Rate Scan?"=w883, "Vin Rate Scan"=w882, "Limits Rate Scan.High"=w864, "Limits Rate Scan.Low"=w863, "Test Rate Scan Adders?"=w881, "Vin Rate Adders"=w880, "Limits Rate Scan adders.High"=w840, "Limits Rate Scan adders.Low"=w839, "Test offset analog?"=w879, "Lim Offset Analog.Max Analog"=w862, "Lim Offset Analog.Min Analog"=w861, "Test offset digital?"=w878, "Lim offset Dig.Max Dig"=w877) -> (w872:T5)
        }
        n404 = local read "VGA"() -> (w817:T14)
        n405 = property on="VALUES VGA" class="Tbl (strict)"() -> ("Row Headers[]"=w814:string[])  [unwired: 2 in, 2 out]
        n406 = local read "Config Rigol DP832"() -> (w816:T13)
        n407 = local read "VISA Rigol DP832"() -> (w815:refnum<visa-resource-name>)
        n408 = Unbundle By Name(w817) -> ("VALUES VGA"=w830:string[][], "TIME VGA.PULSE WIDTH"=w829:u16, "TIME VGA.FRECUENCY PULSE"=w828:dbl)
        n409 = Fract/Exp String To Number(string=w814) -> (number=w836:dbl[])  [unwired: 3 in, 1 out]
        n410 = Divide(x=w836, y=1000.0) -> (x/y=w835:dbl[])
        n411 = Index Array(array=w830, index (col) #1=1 ("disabled index (col)"), index (col) #2=0 ("index (col)")) -> (element #1=w833:string[], element #2=w831:string[])  [unwired: 2 in]
        n412 = Fract/Exp String To Number(string=w833) -> (number=w834:dbl[])  [unwired: 3 in, 1 out]
        n413 = Decimal String To Number(string=w831) -> (number=w832:i32[])  [unwired: 2 in, 1 out]
        n414 = Bundle By Name(cluster=w822, "Config HW.Config Rigol DP832"=w816, "Config HW.VISA Rigol DP832"=w815, "Config HW.CTA Test#"="CTA Board", "Config VGA.Theoretical Voltage"=w835, "Config VGA.Real Voltage"=w834, "Config VGA.VGA Gain"=w832, "Config VGA.Pulse Width"=w829, "Config VGA.Frecuency Pulse"=w828, "Config Test"=w838) -> (w821:T1)
      }
    }
  }
  n415 = flat-sequence {
    tunnel: w1 -> [_]
    frame #0 {
      n416 = local read "Path Config file"() -> (→"Path out":path)
    }
  }
